vi "运维调试_总磷.vi"() -> ()   [LabVIEW 2016, in "斯坦道仪器.lvlib"]
uses:
  <vilib>/Utility/miscctls.llb/LVPointTypeDef.ctl
  <vilib>/Utility/config.llb/NI_LVConfig.lvlib
panel:
  in  "质控参数设置":bool
  out "字符串":string
  in  "总磷自动测试量程配置":T1
  out "温度2":sgl
  out "温度1":sgl
  out "ADC":sgl
  out "固件版本号":string
  in  "数组":string[](array[string])
  in  "备用系数写入":bool
  in  "备用系数读取":bool
  in  "备用系数":T2
  in  "量程切换阈值写入":bool
  in  "量程切换阈值读取":bool
  in  "量程切换阈值":cluster{"阈值":dbl, "标液浓度":dbl}
  in  "参数下拉列表":enum16{"总磷", "总氮"}(ring)
  in  "量程下拉列表":enum16{"低量程", "高量程"}(ring)
  in  "测量模式下拉列表":enum16{"水样测量", "空白核查", "跨度核查", "标样核查", "加标回收"}(ring)
  in  "公式":cluster{"X^2":dbl, "X":dbl, "b":dbl}
  in  "写公式":bool
  in  "读公式":bool
  in  "精度":dbl=4.0
  in  "样品5 F0":dbl
  in  "样品5 F1":dbl
  in  "样品4 F1":dbl
  in  "样品4 F0":dbl
  in  "样品3 F0":dbl
  in  "样品3 F1":dbl
  in  "样品2 F0":dbl
  in  "样品2 F1":dbl
  in  "样品1 F1":dbl
  in  "样品1 F0":dbl
  in  "method":u16(ring) items=["最小二乘", "最小绝对残差", "Bisquare"]
  in  "模型":enum32{"线性", "多项式"}(ring)
  out "r^2":dbl format="%.7g"
  out "拟合公式":string
  in  "样品2启用":bool
  in  "样品5启用":bool
  in  "样品4启用":bool
  in  "样品3启用":bool
  in  "样品1启用":bool
  in  "标液浓度5":dbl
  in  "测量吸光度5":dbl
  in  "标液浓度4":dbl
  in  "测量吸光度4":dbl
  in  "标液浓度3":dbl
  in  "测量吸光度3":dbl
  in  "标液浓度2":dbl
  in  "测量吸光度2":dbl
  in  "测量吸光度1":dbl
  in  "标液浓度1":dbl
  out "XY图":cluster{"X Values":dbl[], "Y Values":dbl[]}[](graph)
  in  "返回":bool
  in  "设置":bool
  out "序列号":string="序列号"
  out "总磷测量数据":T3(xcontrol)
  out "集成报警信息":string
  out "定时启动":bool
  out "总磷总氮运行状态":T4(xcontrol)
  in  "停止":bool
  in  "手动启动":bool
  in  "单步测试":bool
  in  "总磷氨氮调试":u16[](xcontrol)
  out "F3":sgl format="%#.6f"
  out "F2":sgl format="%#.6f"
  out "F1":sgl format="%#.6f"
  out "F0":sgl format="%#.6f"
  out "多列列表框":i32(listbox)
  # "参数设置"
  # "标液浓度"
  # "F0"
  # "F1"
  # "吸光值显示"
  # "样品一"
  # "辅\n助\n计\n算\n区"
  # "样品二"
  # "样品三"
  # "样品四"
  # "样品五"
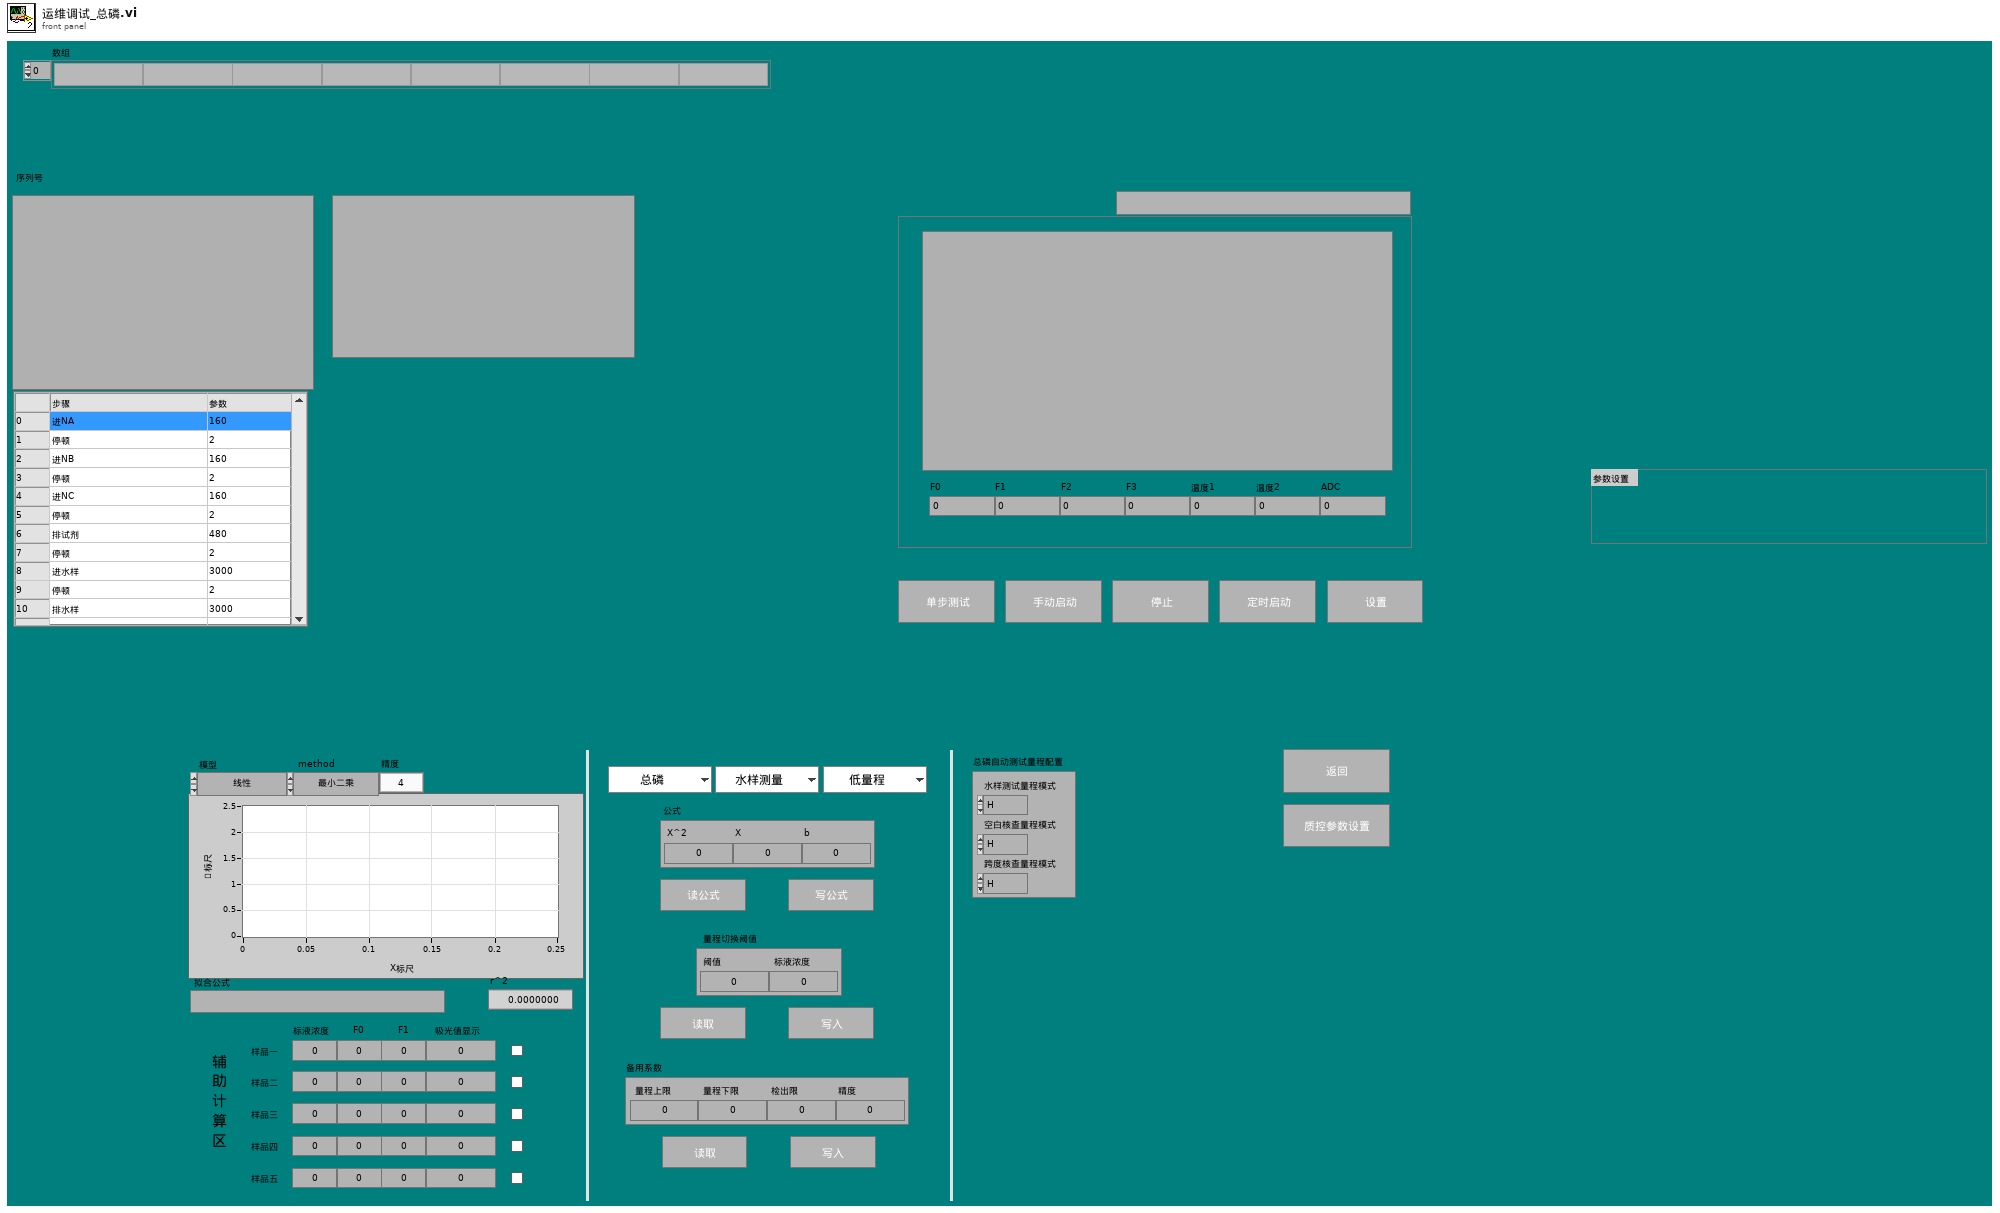
[diagram p1: front panel]
types:
  T1 = cluster{"水样测试量程模式":enum16{"H", "L", "AUTO"}, "空白核查量程模式":enum16{"H", "L", "AUTO"}, "跨度核查量程模式":enum16{"H", "L", "AUTO"}}
  T2 = cluster{"量程上限":dbl, "量程下限":dbl, "检出限":dbl, "精度":dbl}
  T3 = cluster{"flowid":u16, "测量精度":u16, "测量数据区":cluster{"因子编码":u32, "单位":u16, "标样参考值":sgl, "水样数据时间":timestamp, "水样实测值":sgl, "水样数据标识":string, "标样数据时间":timestamp, "标样实测值":sgl, "标样数据标识":string, "空白数据时间":timestamp, "空白实测值":sgl, "空白数据标识":string, "零点核查数据时间":timestamp, "零点核查实测值":sgl, "零点核查数据标识":string, "跨度核查数据时间":timestamp, "跨度核查实测值":sgl, "跨度核查数据标识":string, "加标回收数据时间":timestamp, "加标回收实测值":sgl, "加标回收数据标识":string, "平行样数据时间":timestamp, "平行样实测值":sgl, "平行样数据标识":string, "F0":sgl, "F1":sgl, "F2":sgl, "F3":sgl, "F4":sgl, "F5":sgl, "F6":sgl, "F7":sgl, "温度":sgl, "湿度":sgl, "X值":sgl}}
  T4 = cluster{"系统时间":timestamp, "工作状态":enum16{"空闲", "水样测试", "标样核查", "零点核查", "跨度核查", "空白测试", "平行样测试", "加标回收", "空白校准", "标样校准", "初始化（清洗）"}, "测量模式":enum16{"待机", "连续模式", "周期模式", "定点模式", "受控模式", "手动模式"}, "告警代码":enum16{"无告警", "缺试剂告警", "缺水样告警", "缺蒸馏水告警", "缺标液告警", "仪表漏液告警", "标定异常告警", "超量程告警", "加热异常", "低试剂预警", "超上限告警", "超下限告警", "仪表内部其他异常", "滴定异常告警", "电极异常告警", "量程切换告警", "参数设置告警", "PH电极电位异常", "电导率电极异常", "浊度光度异常", "溶解氧电极异常", "溶解氧光强异常", "温度异常告警", "PH异常告警", "溶解氧异常告警", "电导率异常告警", "浊度异常告警", "叶绿素异常告警", "藻密度异常告警", "蓝绿藻异常告警", "ORP异常告警", "氨氮异常告警", "清洁刷异常告警", "SD卡异常告警", "蓝牙异常告警", "Wifi异常告警", "流程异常告警"}, "故障代码":enum16{"无故障", "电机故障", "温度故障", "通讯故障", "滴定故障"}, "日志代码":u16, "软件版本":u16, "F0":sgl, "F1":sgl, "F2":sgl, "F3":sgl, "T":sgl, "H":sgl, "id":u16, "flowid":u16, "量程":u16, "总磷控温温度1":sgl, "营养盐控温温度2":sgl, "ADC":sgl}
  T5 = cluster{"站号":u16, "量程切换":enum32{"H", "L", "AUTO"}, "控制命令":enum16{"启动测量", "标样核查", "零点核查", "跨度核查", "空白测试", "平行样测试", "加标回收", "空白校准", "标样校准", "初始化（清洗）", "停止测试", "仪器重启", "校时", "模式设置", "测量间隔设置"}, "模式设置":enum16{"待机", "连续模式", "周期模式", "定点模式", "受控模式", "手动模式"}, "测量间隔":u16}
  T6 = enum16{"启动测量", "标样核查", "零点核查", "跨度核查", "空白测试", "平行样测试", "加标回收", "空白校准", "标样校准", "初始化（清洗）", "停止测试", "仪器重启", "校时", "模式设置", "测量间隔设置"}
  T7 = cluster{"仪器测试类型":enum16{"水样测试", "标样核查", "空白测试", "跨度核查"}, "周期设置类型":enum16{"定点启动", "间隔启动"}, "定时功能启用":bool, "定时间隔":dbl, "24H周期设置":bool[]}
  T8 = enum32{"Bad", "Idle", "Run top level", "Running"}
  T9 = typedef "LVDateTimeRec.ctl" = cluster{"秒数的小数部分":dbl, "秒":i32, "分":i32, "时":i32, "日":i32, "月":i32, "年":i32, "天数（周）":i32, "天数（年）":i32, "DST":i32}
  T10 = typedef "LVPointTypeDef.ctl" = cluster{"Horizontal":i16, "Vertical":i16}
  T11 = cluster{"因子编码":u32, "单位":u16, "标样参考值":sgl, "水样数据时间":timestamp, "水样实测值":sgl, "水样数据标识":string, "标样数据时间":timestamp, "标样实测值":sgl, "标样数据标识":string, "空白数据时间":timestamp, "空白实测值":sgl, "空白数据标识":string, "零点核查数据时间":timestamp, "零点核查实测值":sgl, "零点核查数据标识":string, "跨度核查数据时间":timestamp, "跨度核查实测值":sgl, "跨度核查数据标识":string, "加标回收数据时间":timestamp, "加标回收实测值":sgl, "加标回收数据标识":string, "平行样数据时间":timestamp, "平行样实测值":sgl, "平行样数据标识":string, "F0":sgl, "F1":sgl, "F2":sgl, "F3":sgl, "F4":sgl, "F5":sgl, "F6":sgl, "F7":sgl, "温度":sgl, "湿度":sgl, "X值":sgl}
  T12 = enum16{"空闲", "水样测试", "标样核查", "零点核查", "跨度核查", "空白测试", "平行样测试", "加标回收", "空白校准", "标样校准", "初始化（清洗）"}
  T13 = cluster{"启动模式":enum16{"标液测量", "水样测量", "零液测量", "盲样测量", "加标回收"}, "启动参数":u16, "量程":enum16{"低量程", "高量程"}}
  T14 = cluster{"时间标识":timestamp, "设备":string, "日志信息":string, "流程参数":string}
  T15 = cluster{"时间标识":timestamp, "设备":string, "日志信息":string}
  T16 = enum16{"无告警", "缺试剂告警", "缺水样告警", "缺蒸馏水告警", "缺标液告警", "仪表漏液告警", "标定异常告警", "超量程告警", "加热异常", "低试剂预警", "超上限告警", "超下限告警", "仪表内部其他异常", "滴定异常告警", "电极异常告警", "量程切换告警", "参数设置告警", "PH电极电位异常", "电导率电极异常", "浊度光度异常", "溶解氧电极异常", "溶解氧光强异常", "温度异常告警", "PH异常告警", "溶解氧异常告警", "电导率异常告警", "浊度异常告警", "叶绿素异常告警", "藻密度异常告警", "蓝绿藻异常告警", "ORP异常告警", "氨氮异常告警", "清洁刷异常告警", "SD卡异常告警", "蓝牙异常告警", "Wifi异常告警", "流程异常告警"}
  T17 = typedef "LVRowAndColumnUnsignedTypeDef.ctl" = cluster{"Row":u32, "Column":u32}
  T18 = typedef "NI_LVConfig.lvlib/Config Data RefNum.ctl" = refnum<k1>
  T19 = cluster{"XY图":cluster{"X Values":dbl[], "Y Values":dbl[]}[], "标液浓度1":dbl, "测量吸光度1":dbl, "测量吸光度2":dbl, "标液浓度2":dbl, "测量吸光度3":dbl, "标液浓度3":dbl, "测量吸光度4":dbl, "标液浓度4":dbl, "测量吸光度5":dbl, "标液浓度5":dbl, "样品1启用":bool, "样品3启用":bool, "样品4启用":bool, "样品5启用":bool, "样品2启用":bool, "拟合公式":string, "r^2":dbl, "模型":enum32{"线性", "多项式"}, "method":u16, "样品1 F0":dbl, "样品1 F1":dbl, "样品2 F1":dbl, "样品2 F0":dbl, "样品3 F1":dbl, "样品3 F0":dbl, "样品4 F0":dbl, "样品4 F1":dbl, "样品5 F1":dbl, "样品5 F0":dbl, "精度":dbl}
  T20 = cluster{"跨度值":dbl, "零点标准液浓度":dbl, "跨度标准液浓度":dbl, "标准液标准浓度":dbl}
  T21 = cluster{"确定":bool, "跨度值":dbl, "零点标准液浓度":dbl, "跨度标准液浓度":dbl, "标准液标准浓度":dbl}
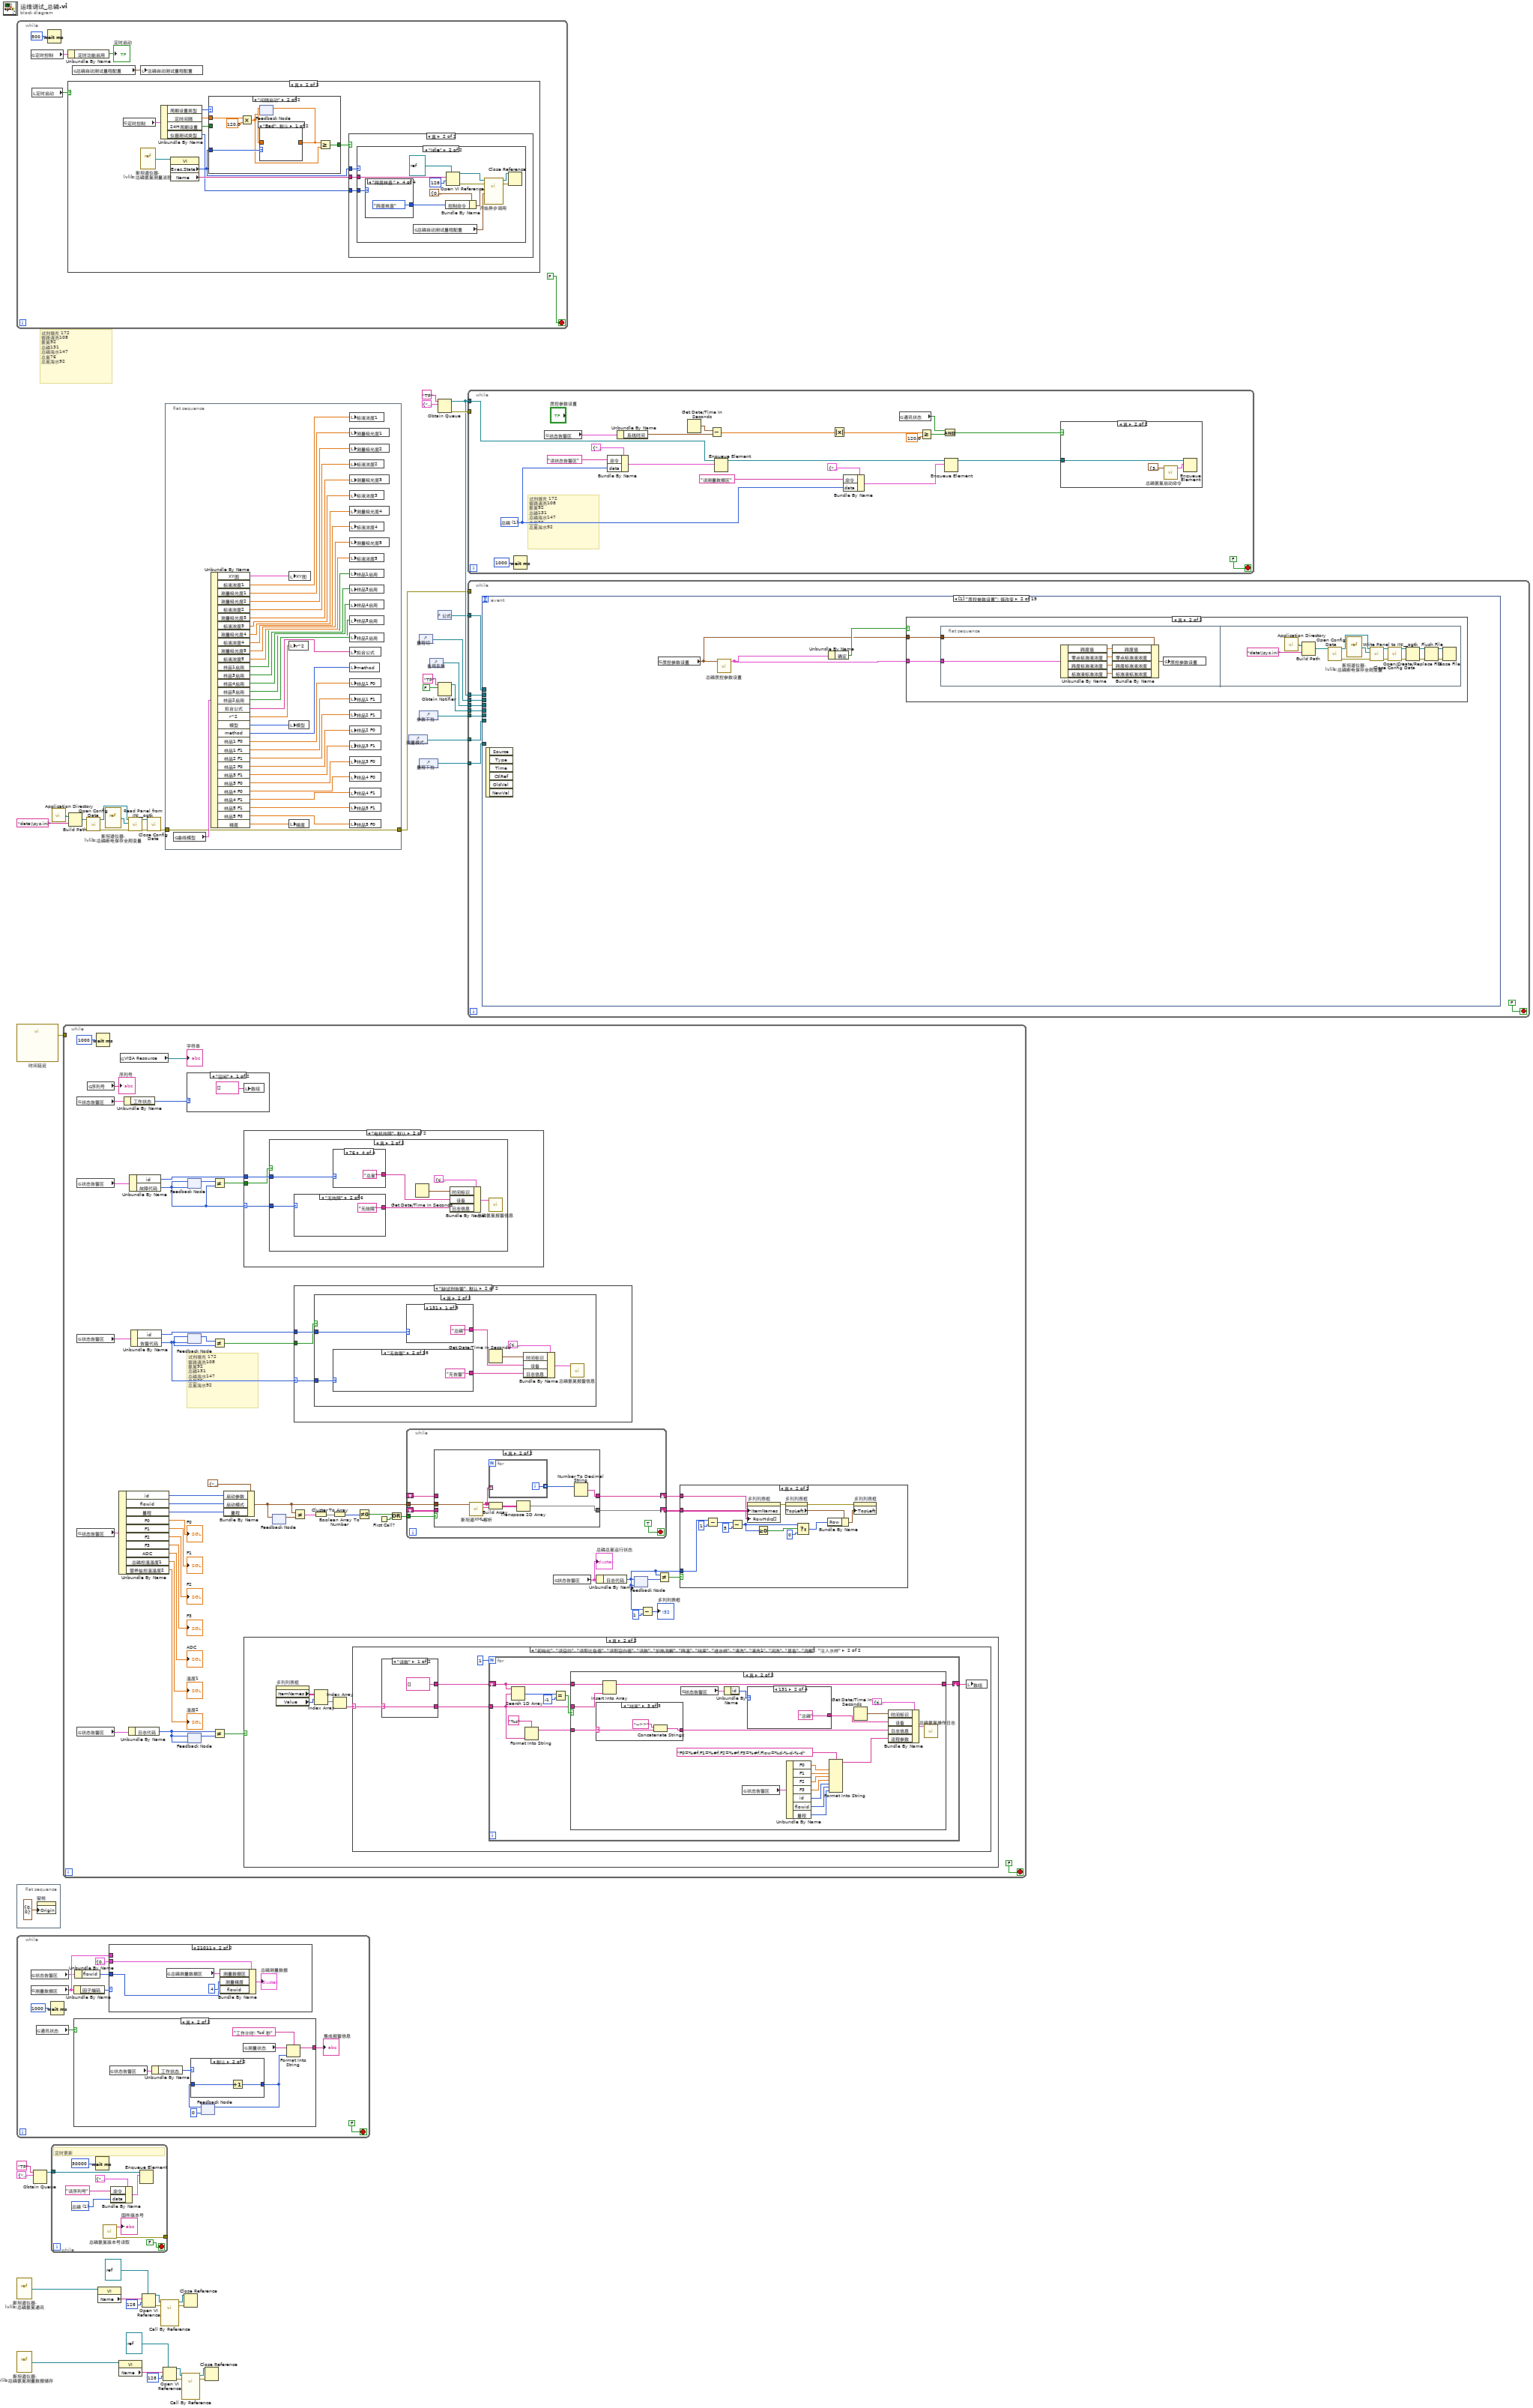
[diagram p0: block diagram]
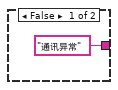
[diagram p2: hidden frame]
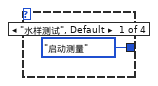
[diagram p8: hidden frame]
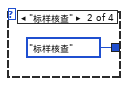
[diagram p9: hidden frame]
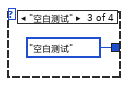
[diagram p10: hidden frame]
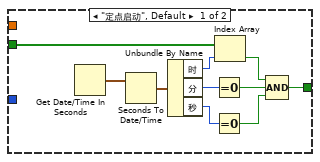
[diagram p11: hidden frame]
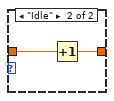
[diagram p12: hidden frame]
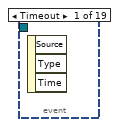
[diagram p13: hidden frame]
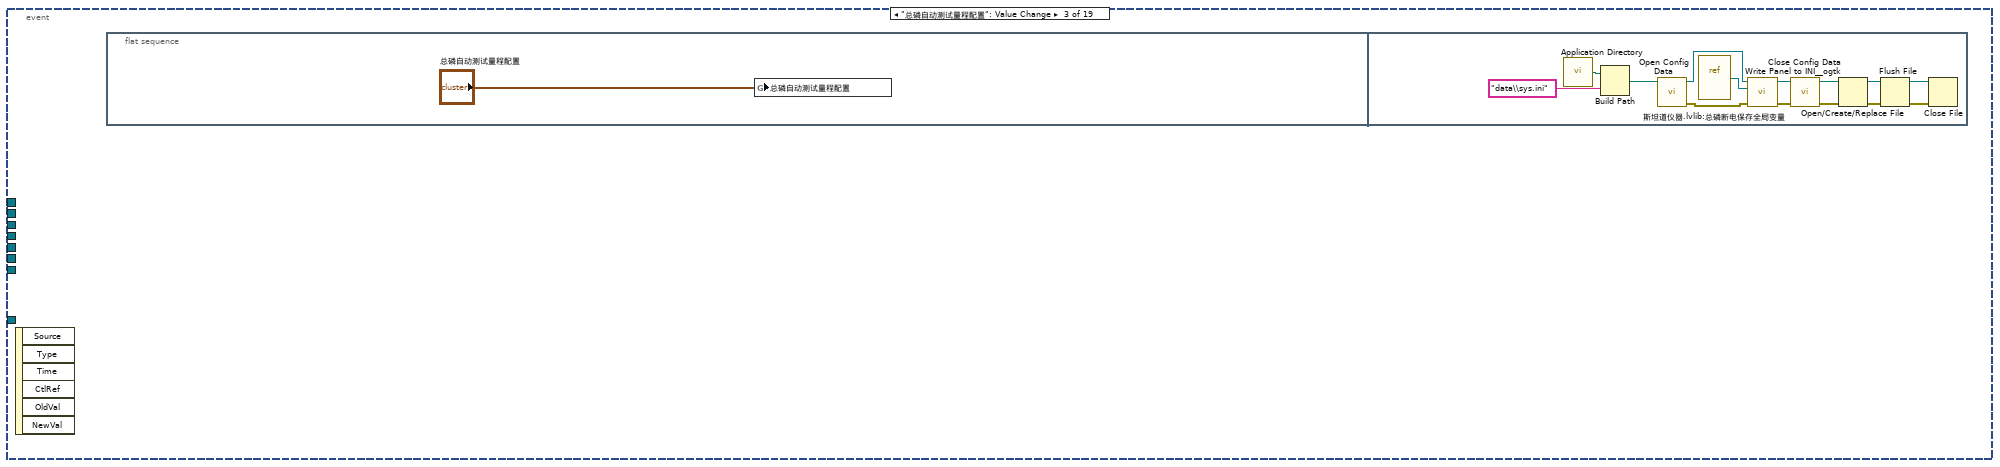
[diagram p15: hidden frame]
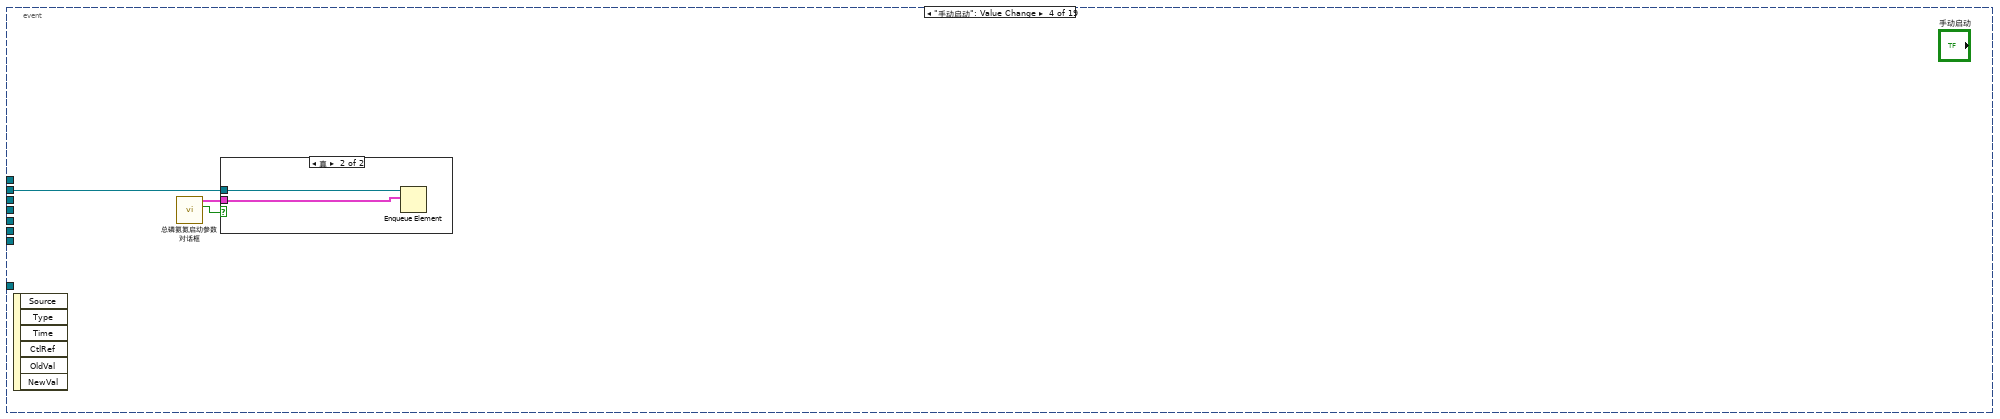
[diagram p16: hidden frame]
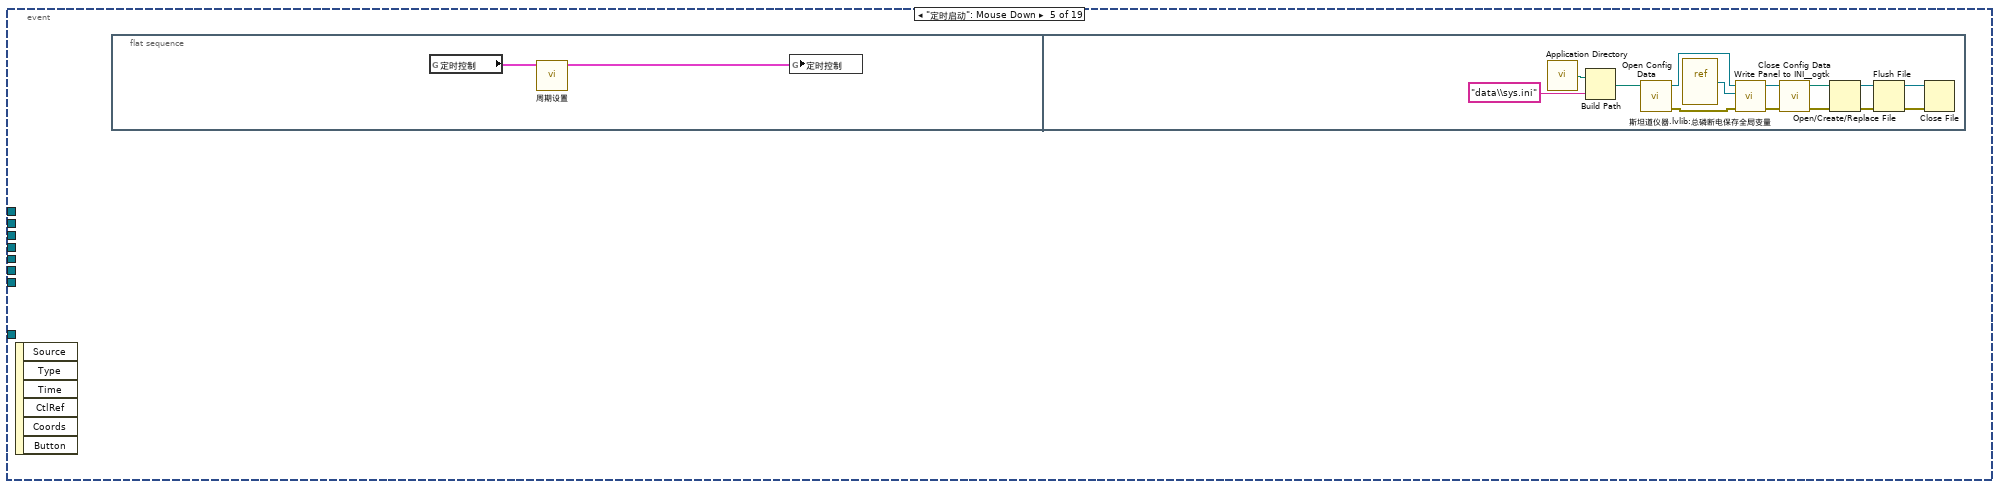
[diagram p18: hidden frame]
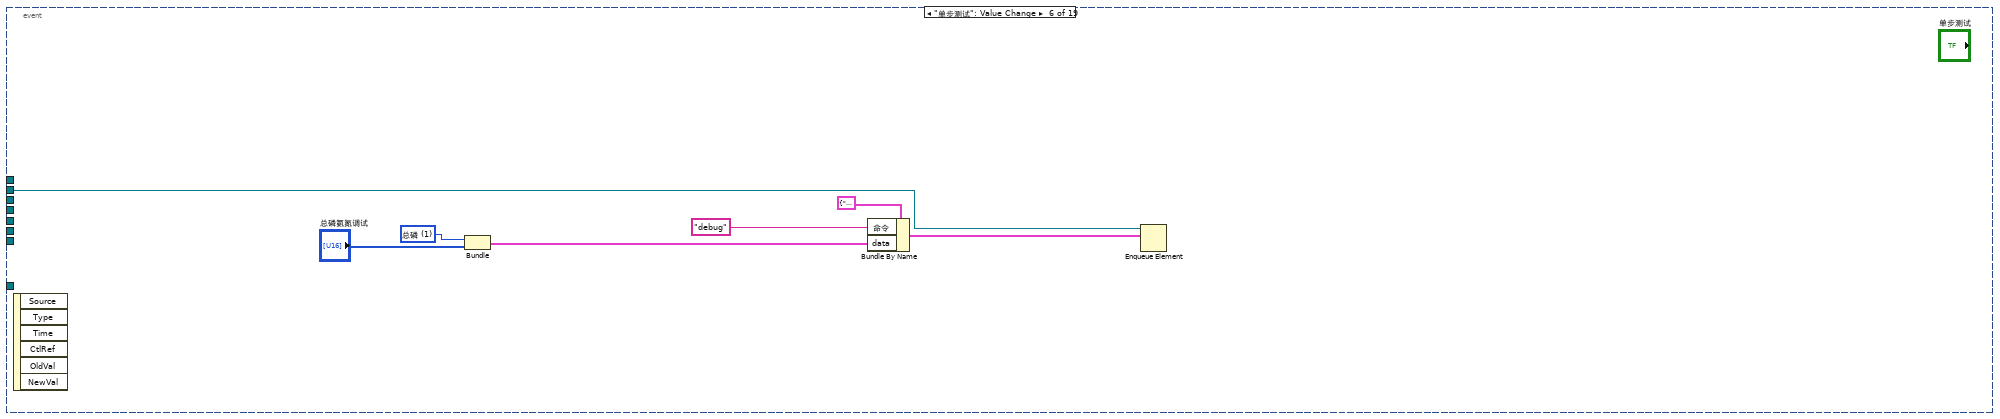
[diagram p19: hidden frame]
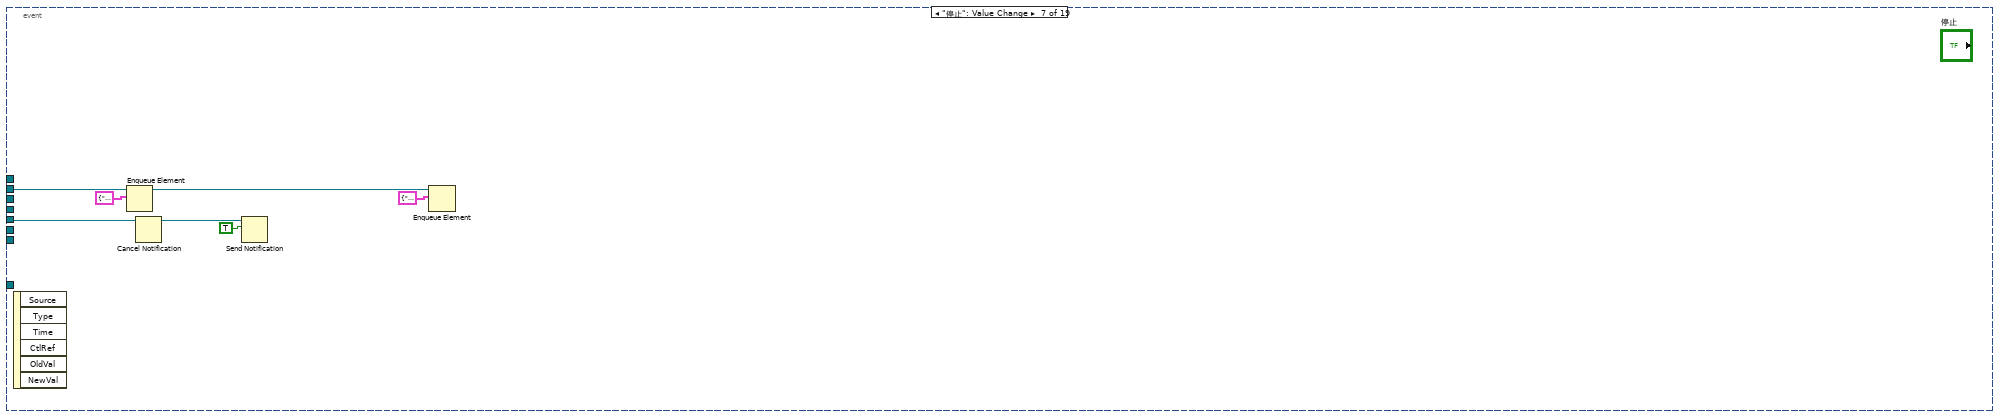
[diagram p20: hidden frame]
diagram:
  # "试剂填充 172 \n管路清洗108\n氨氮92\n总磷131\n总磷海水147\n总氮76\n总氮海水92"
  n1 = while {
    stop <- FALSE stop-if-true
    n2 = global read "总磷断电保存全局变量.vi" "定时控制"() -> (w46:T7)
    n3 = local read "定时启动"() -> (w47:bool)
    n4 = Wait (ms)(milliseconds to wait=u32 500 ("等待时间（毫秒）")) -> ()  [unwired: 1 out]
    n5 = Unbundle By Name(w46) -> ("定时功能启用"=→"定时启动":bool)
    n6 = case shown="真" w47 {
      frame False {
      }
      frame True {
        n7 = global read "总磷断电保存全局变量.vi" "定时控制"() -> (w51:T7)
        n8 = vi-ref "斯坦道仪器.lvlib:总磷氨氮测量流程.vi"() -> (w55:refnum<vi>)
        n9 = Unbundle By Name(w51) -> ("周期设置类型"=w58:enum16{"定点启动", "间隔启动"}, "定时间隔"=w57:dbl, "24H周期设置"=w56:bool[], "仪器测试类型"=w52:enum16{"水样测试", "标样核查", "空白测试", "跨度核查"})
        n10 = property class="VI"(reference=w55) -> ("Exec.State"=w50:T8, "Name"=w54:string)  [unwired: 1 in, 2 out]
        n11 = case shown="\"间隔启动\"" w58 {
          tunnel: w57 -> [_ w91]
          tunnel: w56 -> [w87 _]
          tunnel: w50 -> [_ w94]
          tunnel: [w86 w89] -> w53
          frame "定点启动", Default {
            n12 = Get Date/Time In Seconds() -> (seconds since 1Jan1904=w85:timestamp)
            n13 = Seconds To Date/Time(time stamp (now)=w85) -> (date time rec=w84:T9)  [unwired: 1 in]
            n14 = Unbundle By Name(w84) -> ("时"=w83:i32, "分"=w81:i32, "秒"=w82:i32)
            n15 = Equal To 0?(x=w81) -> (x = 0?=w79:bool)
            n16 = Equal To 0?(x=w82) -> (x = 0?=w78:bool)
            n17 = Index Array(array=w87, index=w83) -> (element=w80:bool)
            n18 = Compound Arithmetic op=AND ("复合运算")(w80, w79, w78) -> (w86:bool)
          }
          frame "间隔启动" {
            n19 = Multiply(x=w91, y=120.0) -> (x*y=w88:dbl)
            n20 = feedback #1(w88) -> (w93:dbl)
            n21 = case shown="\"Bad\", 默认" w94 {
              tunnel: w93 -> [_ w96]
              tunnel: [_ w95] -> w92
              frame "Bad", Default {
              }
              frame "Idle" {
                n22 = Increment(x=w96) -> (x+1=w95:dbl)
              }
            }
            n23 = feedback-in #1(w92) -> ()
            n24 = Greater Or Equal?(x=w92, y=w88) -> (x >= y?=w89:bool)
          }
        }
        n25 = case shown="真" w53 {
          tunnel: w54 -> [_ w61]
          tunnel: w52 -> [_ w60]
          tunnel: w50 -> [_ w59]
          frame False {
          }
          frame True {
            n26 = case shown="\"Idle\"" w59 {
              tunnel: w61 -> [_ w69]
              tunnel: w60 -> [_ w65]
              frame "Bad", Default {
              }
              frame "Idle" {
                n27 = case shown="\"跨度核查\"" w65 {
                  tunnel: [T6."启动测量" ("控制命令") T6."标样核查" ("控制命令") T6."空白测试" ("控制命令") T6."跨度核查" ("控制命令")] -> w64
                  frame "水样测试", Default {
                  }
                  frame "标样核查" {
                  }
                  frame "空白测试" {
                  }
                  frame "跨度核查" {
                  }
                }
                n28 = global read "总磷断电保存全局变量.vi" "总磷自动测试量程配置"() -> (w62:T1)
                n29 = Bundle By Name(cluster=T5 {"站号"=0, "量程切换"=enum."H", "控制命令"=enum."启动测量", "模式设置"=enum."待机", "测量间隔"=0} ("参数"), "控制命令"=w64) -> (w66:T5)
                n30 = Open VI Reference(type specifier VI Refnum (for type only)=refnum<vi> refnum, vi path=w69, options=128 ("选项")) -> (vi reference=w70:refnum<vi>, error out=w71:errorcluster)  [unwired: 3 in]
                n31 = call-by-ref "开始异步调用"(reference=w70, error in=w71, "量程模式"=w62, "参数"=w66) -> (reference out=w72:refnum<vi>, error out=w73:errorcluster)  [unwired: 10 in]
                n32 = Close Reference(reference=w72, error in (no error)=w73) -> ()  [unwired: 1 out]
              }
            }
          }
        }
      }
    }
    n33 = global read "总磷断电保存全局变量.vi" "总磷自动测试量程配置"() -> (w44:T1)
    n34 = local write "总磷自动测试量程配置"(w44) -> ()
  }
  n35 = call "时间延迟"() -> ("error out"=w17:errorcluster)  [unwired: 11 in]
  n36 = flat-sequence {
    frame #0 {
      n37 = property on="窗格" class="Pane"("Origin"=T10 {"Horizontal"=0, "Vertical"=0} ("原点")) -> ()  [unwired: 2 in, 2 out]
    }
  }
  n38 = while {
    stop <- FALSE stop-if-true
    n39 = global read "VAR总磷氨氮全局变量.vi" "状态告警区"() -> (w100:T4)
    n40 = global read "VAR总磷氨氮全局变量.vi" "测量数据区"() -> (w104:T11)
    n41 = global read "VAR总磷氨氮全局变量.vi" "通讯状态"() -> (w102:bool)
    n42 = Wait (ms)(milliseconds to wait=u32 1000 ("等待时间（毫秒）")) -> ()  [unwired: 1 out]
    n43 = Unbundle By Name(w104) -> ("因子编码"=w103:u32)
    n44 = case shown="真" w102 {
      tunnel: ["通讯异常" ("集成报警信息") w109] -> w101
      frame False {
      }
      frame True {
        n45 = global read "VAR总磷氨氮全局变量.vi" "状态告警区"() -> (w115:T4)
        n46 = Unbundle By Name(w115) -> ("工作状态"=w114:T12)
        n47 = feedback #2(0) -> (w112:i32)
        n48 = case shown="默认" w114 {
          tunnel: w112 -> [_ w117]
          tunnel: [_ w116] -> w110
          frame "空闲" {
          }
          frame Default {
            n49 = Increment(x=w117) -> (x+1=w116:i32)
          }
        }
        n50 = feedback-in #2(w110) -> ()
        n51 = global read "VAR总磷氨氮全局变量.vi" "测量状态"() -> (w108:string)
        n52 = Format Into String(format string="工作计时: %d 秒" ("格式字符串"), initial string=w108, w110) -> (resulting string=w109:string)  [unwired: 1 in, 1 out]
      }
    }
    "集成报警信息" <- w101
    n53 = Unbundle By Name(w100) -> ("flowid"=w99:u16)
    n54 = case shown="21011" w103 {
      tunnel: w104 -> [_ _]
      tunnel: w99 -> [_ w120]
      tunnel: T3 {"flowid"=0, "测量精度"=0, "测量数据区"={"因子编码"=0, "单位"=0, "标样参考值"=0.0, "水样数据时间"=timestamp(0 s since 1904-01-01), "水样实测值"=0.0, "水样数据标识"="", "标样数据时间"=timestamp(0 s since 1904-01-01), "标样实测值"=0.0, "标样数据标识"="", "空白数据时间"=timestamp(0 s since 1904-01-01), "空白实测值"=0.0, "空白数据标识"="", "零点核查数据时间"=timestamp(0 s since 1904-01-01), "零点核查实测值"=0.0, "零点核查数据标识"="", "跨度核查数据时间"=timestamp(0 s since 1904-01-01), "跨度核查实测值"=0.0, "跨度核查数据标识"="", "加标回收数据时间"=timestamp(0 s since 1904-01-01), "加标回收实测值"=0.0, "加标回收数据标识"="", "平行样数据时间"=timestamp(0 s since 1904-01-01), "平行样实测值"=0.0, "平行样数据标识"="", "F0"=0.0, "F1"=0.0, "F2"=0.0, "F3"=0.0, "F4"=0.0, "F5"=0.0, "F6"=0.0, "F7"=0.0, "温度"=0.0, "湿度"=0.0, "X值"=0.0}} ("总氮测量数据") -> [_ w119]
      frame Default {
      }
      frame 21011 {
        n55 = global read "VAR总磷氨氮全局变量.vi" "总磷测量数据区"() -> (w118:T11)
        n56 = Bundle By Name(cluster=w119, "测量数据区"=w118, "测量精度"=u16 4, "flowid"=w120) -> (→"总磷测量数据":T3)
      }
    }
  }
  n57 = vi-ref "斯坦道仪器.lvlib:总磷氨氮通讯.vi"() -> (w39:refnum<vi>)
  n58 = vi-ref "斯坦道仪器.lvlib:总磷氨氮测量数据储存.vi"() -> (w31:refnum<vi>)
  n59 = Obtain Queue(name (unnamed)="TP" ("名称（未命名）"), element data type=cluster{"命令":string, "data":variant} {"命令"="", "data"=variant}) -> (queue out=w14:refnum<queue>)  [unwired: 3 in, 2 out]
  n60 = while {
    tunnel: w14 -> [w128]
    tunnel: [w124] -> _
    stop <- FALSE stop-if-true
    w125 = u16 1 items=["总磷"=1, "总氮"=2, "氨氮"=3] ("站号")
    # "定时更新"
    n61 = Wait (ms)(milliseconds to wait=u32 30000 ("等待时间（毫秒）")) -> ()  [unwired: 1 out]
    n62 = call "总磷氨氮版本号读取.vi"() -> ("error out"=w124:errorcluster, "固件版本号"=→"固件版本号":string)  [unwired: 10 in]
    n63 = Bundle By Name(cluster=cluster{"命令":string, "data":variant} {"命令"="", "data"=variant} ("元素"), "命令"="读序列号", "data"=w125) -> (w127:cluster{"命令":string, "data":variant})
    n64 = Enqueue Element(queue=w128, element=w127) -> ()  [unwired: 2 in, 3 out]
  }
  n65 = call <vilib>:"Application Directory.vi"() -> ("Application Directory"=w3:path)
  n66 = while {
    tunnel: w17 -> [_]
    stop <- FALSE stop-if-true
    # "试剂填充 172 \n管路清洗108\n氨氮92\n总磷131\n总磷海水147\n总氮76\n总氮海水92"
    n67 = global read "VAR总磷氨氮全局变量.vi" "状态告警区"() -> (w144:T4)
    n68 = global read "VAR总磷氨氮全局变量.vi" "状态告警区"() -> (w149:T4)
    n69 = global read "VAR总磷氨氮全局变量.vi" "状态告警区"() -> (w154:T4)
    n70 = global read "VAR总磷氨氮全局变量.vi" "状态告警区"() -> (w166:T4)
    n71 = global read "VAR总磷氨氮全局变量.vi" "状态告警区"() -> (w141:T4)
    n72 = global read "VAR总磷氨氮全局变量.vi" "序列号"() -> (→"序列号":string)
    n73 = Wait (ms)(milliseconds to wait=u32 1000 ("等待时间（毫秒）")) -> ()  [unwired: 1 out]
    n74 = Unbundle By Name(w166) -> ("id"=w163:u16, "flowid"=w165:u16, "量程"=w164:u16, "F0"=→"F0":sgl, "F1"=→"F1":sgl, "F2"=→"F2":sgl, "F3"=→"F3":sgl, "ADC"=→"ADC":sgl, "总磷控温温度1"=→"温度1":sgl, "营养盐控温温度2"=→"温度2":sgl)
    n75 = global read "VAR总磷氨氮全局变量.vi" "VISA Resource"() -> (→"字符串":refnum<visa-resource-name>)
    n76 = Unbundle By Name(w144) -> ("工作状态"=w143:T12)
    n77 = Unbundle By Name(w141) -> ("日志代码"=w140:u16)
    n78 = Unbundle By Name(w149) -> ("id"=w148:u16, "故障代码"=w145:enum16{"无故障", "电机故障", "温度故障", "通讯故障", "滴定故障"})
    n79 = Unbundle By Name(w154) -> ("id"=w153:u16, "告警代码"=w150:T16)
    n80 = case shown="\"空闲\"" w143 {
      frame "空闲" {
        n81 = local write "数组"(string[] [] ("数组")) -> ()
      }
      frame "水样测试", Default {
      }
    }
    n82 = feedback #3(w145) -> (w146:enum16{"无故障", "电机故障", "温度故障", "通讯故障", "滴定故障"})
    n83 = feedback-in #3(w145) -> ()
    n84 = feedback #4(w150) -> (w151:T16)
    n85 = feedback-in #4(w150) -> ()
    n86 = feedback #5(w140) -> (w142:u16)
    n87 = feedback-in #5(w140) -> ()
    n88 = Not Equal?(x=w146, y=w145) -> (x != y?=w147:bool)
    n89 = Not Equal?(x=w151, y=w150) -> (x != y?=w152:bool)
    n90 = Not Equal?(x=w140, y=w142) -> (x != y?=w139:bool)
    n91 = Bundle By Name(cluster=T13 {"启动模式"=enum."加标回收", "启动参数"=1, "量程"=enum."低量程"} ("参数簇"), "启动参数"=w163, "启动模式"=w165, "量程"=w164) -> (w156:T13)
    n92 = case shown="\"电机故障\", 默认" w145 {
      selector: w145 -> [_ w235]
      tunnel: w148 -> [_ w236]
      tunnel: w147 -> [_ w234]
      frame "无故障" {
      }
      frame "电机故障", Default {
        n93 = case shown="真" w234 {
          tunnel: w236 -> [_ w243]
          tunnel: w235 -> [_ w238]
          frame False {
          }
          frame True {
            n94 = case shown="\"无故障\"" w238 {
              selector: w238 -> [w245 _ _ _ _ _]
              tunnel: [w244 "无故障" "电机故障" "温度故障" "通讯故障" "滴定故障"] -> w237
              frame Default {
                n95 = Format Into String(format string="%d" ("格式字符串"), initial string="未知" ("工作状态"), w245) -> (resulting string=w244:string)  [unwired: 1 in, 1 out]
              }
              frame "无故障" {
              }
              frame "电机故障" {
              }
              frame "温度故障" {
              }
              frame "通讯故障" {
              }
              frame "滴定故障" {
              }
            }
            n96 = case shown="76" w243 {
              tunnel: [_ "总磷" ("table输入") "氨氮" ("table输入") "总氮" ("table输入")] -> w239
              frame Default {
              }
              frame 131 {
              }
              frame 92 {
              }
              frame 76 {
              }
            }
            n97 = Get Date/Time In Seconds() -> (seconds since 1Jan1904=w240:timestamp)
            n98 = Bundle By Name(cluster=T15 {"时间标识"=timestamp(0 s since 1904-01-01), "设备"="", "日志信息"=""} ("data in"), "时间标识"=w240, "设备"=w239, "日志信息"=w237) -> (w241:T15)
            n99 = call "总磷氨氮报警信息.vi"("data in"=w241) -> ()  [unwired: 11 in]
          }
        }
      }
    }
    n100 = case shown="真" w139 {
      frame False {
      }
      frame True {
        n101 = property on="多列列表框" class="MCListbox (严格)"() -> ("ItemNames"=w183:string[][], "Value"=w184:i32)  [unwired: 2 in, 2 out]
        n102 = Index Array(array=w183, index (row)=w184) -> (element=w182:string[])  [unwired: 1 in]
        n103 = Index Array(array=w182) -> (element=w181:string)  [unwired: 1 in]
        n104 = case shown="\"初始化\", \"读空白\", \"读取比色值\", \"读取空白值\", \"读数\", \"加热消解\", \"降温\", \"结束\", \"进水样\", \"清洗\", \"清洗1\", \"润洗\", \"显色\", \"消解\", \"注入水样\"" w181 {
          selector: w181 -> [_ w187]
          frame Default {
          }
          frame "初始化", "读空白", "读取比色值", "读取空白值", "读数", "加热消解", "降温", "结束", "进水样", "清洗", "清洗1", "润洗", "显色", "消解", "注入水样" {
            n105 = case shown="\"读数\"" w187 {
              selector: w187 -> [w191 w193]
              tunnel: [w191 w193] -> w186
              tunnel: [string[] [] ("数组") "数组"] -> w185
              frame "读数" {
              }
              frame Default {
              }
            }
            n106 = for {
              N: 1 -> [_]
              tunnel: w186 -> [w195]
              shift-right: [w194] -> w188
              shift-left: w185 -> [w196]
              n107 = Search 1D Array(1D array=w196, element=w195) -> (index of element=w199:i32)  [unwired: 1 in]
              n108 = Format Into String(format string="%s" ("格式字符串"), w195) -> (resulting string=w200:string)  [unwired: 2 in, 1 out]
              n109 = Equal?(x=w199, y=-1) -> (x = y?=w197:bool)
              n110 = case shown="真" w197 {
                tunnel: w200 -> [_ w204]
                tunnel: w196 -> [w202 w208]
                tunnel: w195 -> [_ w207]
                tunnel: [w202 w206] -> w194
                frame False {
                }
                frame True {
                  n111 = case shown="\"结束\"" w204 {
                    selector: w204 -> [w224 w227 w230]
                    tunnel: [w224 w226 w229] -> w203
                    frame Default {
                    }
                    frame "初始化" {
                      n112 = Concatenate Strings("-->>" ("字符串"), w227) -> (w226:string)
                    }
                    frame "结束" {
                      n113 = Concatenate Strings("-->>" ("字符串"), w230) -> (w229:string)
                    }
                  }
                  n114 = Insert Into Array(array=w208, new element=w207) -> (w206:string[])  [unwired: 1 in]
                  n115 = global read "VAR总磷氨氮全局变量.vi" "状态告警区"() -> (w223:T4)
                  n116 = Unbundle By Name(w223) -> ("id"=w222:u16)
                  n117 = global read "VAR总磷氨氮全局变量.vi" "状态告警区"() -> (w218:T4)
                  n118 = case shown="131" w222 {
                    tunnel: [_ "总磷" ("table输入") "氨氮" ("table输入") "总氮" ("table输入")] -> w220
                    frame Default {
                    }
                    frame 131 {
                    }
                    frame 92 {
                    }
                    frame 76 {
                    }
                  }
                  n119 = Unbundle By Name(w218) -> ("F0"=w215:sgl, "F1"=w214:sgl, "F2"=w213:sgl, "F3"=w212:sgl, "id"=w211:u16, "flowid"=w210:u16, "量程"=w209:u16)
                  n120 = Format Into String(format string="F0=%#f,F1=%#f,F2=%#f,F3=%#f,Flow=%d-%-d-%-d" ("格式字符串"), w215, w214, w213, w212, w211, w210, w209) -> (resulting string=w216:string)  [unwired: 2 in, 1 out]
                  n121 = Get Date/Time In Seconds() -> (seconds since 1Jan1904=w219:timestamp)
                  n122 = Bundle By Name(cluster=T14 {"时间标识"=timestamp(0 s since 1904-01-01), "设备"="", "日志信息"="", "流程参数"=""} ("data in"), "时间标识"=w219, "设备"=w220, "日志信息"=w203, "流程参数"=w216) -> (w221:T14)
                  n123 = call "总磷氨氮操作日志.vi"("data in"=w221) -> ()  [unwired: 11 in]
                }
              }
            }
            n124 = local write "数组"(w188) -> ()
          }
        }
      }
    }
    n125 = feedback #6() -> (w172:T13)  [unwired: 1 in]
    n126 = feedback-in #6(w156) -> ()
    n127 = Not Equal?(x=w156, y=w172) -> (x != y?=w173:cluster{"启动模式":bool, "启动参数":bool, "量程":bool})
    n128 = case shown="\"缺试剂告警\", 默认" w150 {
      selector: w150 -> [_ w257]
      tunnel: w153 -> [_ w258]
      tunnel: w152 -> [_ w256]
      frame "无告警" {
      }
      frame "缺试剂告警", Default {
        n129 = case shown="真" w256 {
          tunnel: w258 -> [_ w265]
          tunnel: w257 -> [_ w259]
          frame False {
          }
          frame True {
            n130 = case shown="\"无告警\"" w259 {
              selector: w259 -> [w267 _ _ _ _ _ _ _ _ _ _ _ _ _ _ _ _ _ _ _ _ _ _ _ _ _ _ _ _ _ _ _ _ _ _ _ _ _]
              tunnel: [w266 "无告警" "缺试剂告警" "缺水样告警" "缺蒸馏水告警" "缺标液告警" "仪表漏液告警" "标定异常告警" "超量程告警" "加热异常" "低试剂预警" "超上限告警" "超下限告警" "仪表内部其他异常" "滴定异常告警" "电极异常告警" "量程切换告警" "参数设置告警" "PH电极电位异常" "电导率电极异常" "浊度光度异常" "溶解氧电极异常" "溶解氧光强异常" "温度异常告警" "PH异常告警" "溶解氧异常告警" "电导率异常告警" "浊度异常告警" "叶绿素异常告警" "藻密度异常告警" "蓝绿藻异常告警" "ORP异常告警" "氨氮异常告警" "清洁刷异常告警" "SD卡异常告警" "蓝牙异常告警" "WiFi异常告警" "流程异常告警"] -> w260
              frame Default {
                n131 = Format Into String(format string="%d" ("格式字符串"), initial string="未知" ("工作状态"), w267) -> (resulting string=w266:string)  [unwired: 1 in, 1 out]
              }
              frame "无告警" {
              }
              frame "缺试剂告警" {
              }
              frame "缺水样告警" {
              }
              frame "缺蒸馏水告警" {
              }
              frame "缺标液告警" {
              }
              frame "仪表漏液告警" {
              }
              frame "标定异常告警" {
              }
              frame "超量程告警" {
              }
              frame "加热异常" {
              }
              frame "低试剂预警" {
              }
              frame "超上限告警" {
              }
              frame "超下限告警" {
              }
              frame "仪表内部其他异常" {
              }
              frame "滴定异常告警" {
              }
              frame "电极异常告警" {
              }
              frame "量程切换告警" {
              }
              frame "参数设置告警" {
              }
              frame "PH电极电位异常" {
              }
              frame "电导率电极异常" {
              }
              frame "浊度光度异常" {
              }
              frame "溶解氧电极异常" {
              }
              frame "溶解氧光强异常" {
              }
              frame "温度异常告警" {
              }
              frame "PH异常告警" {
              }
              frame "溶解氧异常告警" {
              }
              frame "电导率异常告警" {
              }
              frame "浊度异常告警" {
              }
              frame "叶绿素异常告警" {
              }
              frame "藻密度异常告警" {
              }
              frame "蓝绿藻异常告警" {
              }
              frame "ORP异常告警" {
              }
              frame "氨氮异常告警" {
              }
              frame "清洁刷异常告警" {
              }
              frame "SD卡异常告警" {
              }
              frame "蓝牙异常告警" {
              }
              frame "Wifi异常告警" {
              }
              frame "流程异常告警" {
              }
            }
            n132 = case shown="131" w265 {
              tunnel: ["总磷" ("table输入") "氨氮" ("table输入") "总氮" ("table输入")] -> w261
              frame 131 {
              }
              frame 92 {
              }
              frame 76, Default {
              }
            }
            n133 = Get Date/Time In Seconds() -> (seconds since 1Jan1904=w262:timestamp)
            n134 = Bundle By Name(cluster=T15 {"时间标识"=timestamp(0 s since 1904-01-01), "设备"="", "日志信息"=""} ("data in"), "时间标识"=w262, "设备"=w261, "日志信息"=w260) -> (w263:T15)
            n135 = call "总磷氨氮报警信息.vi"("data in"=w263) -> ()  [unwired: 11 in]
          }
        }
      }
    }
    n136 = Cluster To Array(cluster=w173) -> (array=w174:bool[])
    n137 = Boolean Array To Number(Boolean array=w174) -> (number=w175:u32)
    n138 = Not Equal To 0?(x=w175) -> (x != 0?=w168:bool)
    n139 = First Call?() -> (First Call?: T/F=w169:bool)
    n140 = Or(x=w168, y=w169) -> (x .or. y?=w167:bool)
    n141 = while {
      tunnel: w167 -> [w316]
      tunnel: w156 -> [w315]
      shift-right: [w314] -> w171
      shift-left: _ -> [w310]
      shift-right: [w313] -> w170
      shift-left: _ -> [w311]
      stop <- TRUE stop-if-true
      n142 = case shown="真" w316 {
        tunnel: [w318 w325] -> w313
        tunnel: [w317 w324] -> w314
        tunnel: w315 -> [_ w319]
        tunnel: w311 -> [w318 _]
        tunnel: w310 -> [w317 _]
        frame False {
        }
        frame True {
          n143 = call "斯坦道XML解析.vi"("参数簇"=w319) -> ("步骤时间"=w320:string[], "步骤名"=w322:string[])  [unwired: 9 in]
          n144 = for {
            tunnel: w322 -> [_] mode=indexing
            tunnel: [w326] -> w323 mode=indexing
            i -> [w326]
          }
          n145 = Build Array(w322, w320) -> (w321:string[][])
          n146 = Transpose 2D Array(2D array=w321) -> (transposed array=w324:string[][])
          n147 = Number To Decimal String(number=w323) -> (decimal integer string=w325:string[])  [unwired: 1 in]
        }
      }
    }
    n148 = global read "VAR总磷氨氮全局变量.vi" "状态告警区"() -> (w157:T4)
    "总磷总氮运行状态" <- w157
    n149 = Unbundle By Name(w157) -> ("日志代码"=w137:u16)
    n150 = feedback-in #7(w137) -> ()
    n151 = feedback #7(w137) -> (w177:u16)
    n152 = Subtract(x=w137, y=1) -> (x-y=→"多列列表框":i32)
    n153 = Not Equal?(x=w137, y=w177) -> (x != y?=w176:bool)
    n154 = case shown="真" w176 {
      tunnel: w137 -> [_ w329]
      tunnel: w171 -> [_ w336]
      tunnel: w170 -> [_ w335]
      frame False {
      }
      frame True {
        n155 = Subtract(x=w329, y=1) -> (x-y=w327:i32)
        n156 = Subtract(x=w327, y=5) -> (x-y=w331:i32)
        n157 = property on="多列列表框" class="MCListbox (严格)"("ItemNames"=w336, "RowHdrs[]"=w335) -> (error out=w337:errorcluster)  [unwired: 2 in, 1 out]
        n158 = Greater Or Equal To 0?(x=w331) -> (x >= 0?=w330:bool)
        n159 = property on="多列列表框" class="MCListbox (严格)"(error in=w337) -> (error out=w338:errorcluster, "TopLeft"=w339:T17)  [unwired: 1 in, 1 out]
        n160 = Select(t=w331, s=w330, f=0) -> (s? t:f=w332:i32)
        n161 = Bundle By Name(cluster=w339, "Row"=w332) -> (w340:T17)
        n162 = property on="多列列表框" class="MCListbox (严格)"(error in=w338, "TopLeft"=w340) -> ()  [unwired: 1 in, 2 out]
      }
    }
  }
  n163 = Build Path(base path=w3, name or relative path="data\\sys.ini" ("名称或相对路径")) -> (appended path=w5:path)
  n164 = call <vilib>:"Open Config Data.vi"("configuration file path"=w5) -> ("error out"=w9:errorcluster, "refnum"=w6:T18)  [unwired: 8 in, 1 out]
  n165 = property class="VI"(reference=w39) -> ("Name"=w38:string)  [unwired: 1 in, 2 out]
  n166 = vi-ref "斯坦道仪器.lvlib:总磷断电保存全局变量.vi"() -> (w7:refnum<vi>)
  n167 = property class="VI"(reference=w31) -> ("Name"=w24:string)  [unwired: 1 in, 2 out]
  n168 = call <userlib>:"Read Panel from INI__ogtk.vi"("error in (no error)"=w9, "VI ref"=w7, "refnum"=w6) -> ("error out"=w10:errorcluster, "refnum out"=w8:T18)  [unwired: 7 in]
  n169 = Open VI Reference(type specifier VI Refnum (for type only)=refnum<vi> refnum, vi path=w38, options=128 ("选项")) -> (vi reference=w36:refnum<vi>, error out=w34:errorcluster)  [unwired: 3 in]
  n170 = call <vilib>:"Close Config Data.vi"("error in (no error)"=w10, "refnum"=w8) -> ("error out"=w2:errorcluster)  [unwired: 8 in, 1 out]
  n171 = call-by-ref "?"(reference=w36, error in=w34) -> (reference out=w32:refnum<vi>, error out=w33:errorcluster)  [unwired: 12 in]
  n172 = Open VI Reference(type specifier VI Refnum (for type only)=refnum<vi> refnum, vi path=w24, options=128 ("选项")) -> (vi reference=w26:refnum<vi>, error out=w28:errorcluster)  [unwired: 3 in]
  n173 = flat-sequence {
    tunnel: w2 -> [w341]
    tunnel: [w341] -> w1
    frame #0 {
      n174 = global read "总磷断电保存全局变量.vi" "曲线模型"() -> (w373:T19)
      n175 = Unbundle By Name(w373) -> ("XY图"=w372:cluster{"X Values":dbl[], "Y Values":dbl[]}[], "标液浓度1"=w371:dbl, "测量吸光度1"=w370:dbl, "测量吸光度2"=w369:dbl, "标液浓度2"=w362:dbl, "测量吸光度3"=w368:dbl, "标液浓度3"=w363:dbl, "测量吸光度4"=w367:dbl, "标液浓度4"=w364:dbl, "测量吸光度5"=w366:dbl, "标液浓度5"=w365:dbl, "样品1启用"=w361:bool, "样品3启用"=w360:bool, "样品4启用"=w359:bool, "样品5启用"=w358:bool, "样品2启用"=w357:bool, "拟合公式"=w356:string, "r^2"=w355:dbl, "模型"=w354:enum32{"线性", "多项式"}, "method"=w353:u16, "样品1 F0"=w352:dbl, "样品1 F1"=w351:dbl, "样品2 F1"=w350:dbl, "样品2 F0"=w349:dbl, "样品3 F1"=w348:dbl, "样品3 F0"=w347:dbl, "样品4 F0"=w346:dbl, "样品4 F1"=w345:dbl, "样品5 F1"=w344:dbl, "样品5 F0"=w343:dbl, "精度"=w342:dbl)
      n176 = local write "XY图"(w372) -> ()
      n177 = local write "r^2"(w355) -> ()
      n178 = local write "模型"(w354) -> ()
      n179 = local write "精度"(w342) -> ()
      n180 = local write "标液浓度1"(w371) -> ()
      n181 = local write "测量吸光度1"(w370) -> ()
      n182 = local write "测量吸光度2"(w369) -> ()
      n183 = local write "标液浓度2"(w362) -> ()
      n184 = local write "测量吸光度3"(w368) -> ()
      n185 = local write "标液浓度3"(w363) -> ()
      n186 = local write "测量吸光度4"(w367) -> ()
      n187 = local write "标液浓度4"(w364) -> ()
      n188 = local write "测量吸光度5"(w366) -> ()
      n189 = local write "标液浓度5"(w365) -> ()
      n190 = local write "样品1启用"(w361) -> ()
      n191 = local write "样品3启用"(w360) -> ()
      n192 = local write "样品4启用"(w359) -> ()
      n193 = local write "样品5启用"(w358) -> ()
      n194 = local write "样品2启用"(w357) -> ()
      n195 = local write "拟合公式"(w356) -> ()
      n196 = local write "method"(w353) -> ()
      n197 = local write "样品1 F0"(w352) -> ()
      n198 = local write "样品1 F1"(w351) -> ()
      n199 = local write "样品2 F1"(w350) -> ()
      n200 = local write "样品2 F0"(w349) -> ()
      n201 = local write "样品3 F1"(w348) -> ()
      n202 = local write "样品3 F0"(w347) -> ()
      n203 = local write "样品4 F0"(w346) -> ()
      n204 = local write "样品4 F1"(w345) -> ()
      n205 = local write "样品5 F1"(w344) -> ()
      n206 = local write "样品5 F0"(w343) -> ()
    }
  }
  n207 = call-by-ref "?"(reference=w26, error in=w28) -> (reference out=w30:refnum<vi>, error out=w29:errorcluster)  [unwired: 12 in]
  n208 = Close Reference(reference=w32, error in (no error)=w33) -> ()  [unwired: 1 out]
  n209 = Close Reference(reference=w30, error in (no error)=w29) -> ()  [unwired: 1 out]
  n210 = control-ref of="测量模式下拉列表"() -> (w21:refnum<vi>)
  n211 = control-ref of="量程切换阈值"() -> (w19:refnum<vi>)
  n212 = control-ref of="参数下拉列表"() -> (w22:refnum<vi>)
  n213 = control-ref of="量程下拉列表"() -> (w23:refnum<vi>)
  n214 = control-ref of="备用系数"() -> (w18:refnum<vi>)
  n215 = control-ref of="公式"() -> (w20:refnum<vi>)
  n216 = Obtain Queue(name (unnamed)="TP" ("名称（未命名）"), element data type=cluster{"命令":string, "data":variant} {"命令"="", "data"=variant}) -> (queue out=w40:refnum<queue>, error out=w41:errorcluster)  [unwired: 3 in, 1 out]
  n217 = Obtain Notifier(name (unnamed)="TP" ("名称（未命名）"), notification data type=FALSE) -> (notifier out=w11:refnum<notifier>)  [unwired: 2 in, 2 out]
  n218 = while {
    tunnel: w40 -> [w389]
    tunnel: w41 -> [_]
    stop <- FALSE stop-if-true
    w376 = u16 1 items=["总磷"=1, "总氮"=2, "氨氮"=3] ("站号")
    # "试剂填充 172 \n管路清洗108\n氨氮92\n总磷131\n总磷海水147\n总氮76\n总氮海水92"
    n219 = Wait (ms)(milliseconds to wait=u32 1000 ("等待时间（毫秒）")) -> ()  [unwired: 1 out]
    n220 = global read "VAR总磷氨氮全局变量.vi" "状态告警区"() -> (w377:T4)
    n221 = Bundle By Name(cluster=cluster{"命令":string, "data":variant} {"命令"="", "data"=variant} ("元素"), "命令"="读状态告警区", "data"=w376) -> (w391:cluster{"命令":string, "data":variant})
    n222 = Unbundle By Name(w377) -> ("系统时间"=w384:timestamp)
    n223 = Get Date/Time In Seconds() -> (seconds since 1Jan1904=w383:timestamp)
    n224 = Subtract(x=w383, y=w384) -> (x-y=w382:dbl)
    n225 = Enqueue Element(queue=w389, element=w391) -> (queue out=w385:refnum<queue>)  [unwired: 2 in, 2 out]
    n226 = Absolute Value(x=w382) -> (abs(x)=w381:dbl)
    n227 = Bundle By Name(cluster=cluster{"命令":string, "data":variant} {"命令"="", "data"=variant} ("元素"), "命令"="读测量数据区", "data"=w376) -> (w387:cluster{"命令":string, "data":variant})
    n228 = global read "VAR总磷氨氮全局变量.vi" "通讯状态"() -> (w374:bool)
    n229 = Greater Or Equal?(x=w381, y=120.0) -> (x >= y?=w379:bool)
    n230 = And(x=w374, y=w379) -> (x .and. y?=w375:bool)
    n231 = Enqueue Element(queue=w385, element=w387) -> (queue out=w378:refnum<queue>)  [unwired: 2 in, 2 out]
    n232 = case shown="真" w375 {
      tunnel: w378 -> [_ w396]
      frame False {
      }
      frame True {
        n233 = call "总磷氨氮启动命令.vi"("参数"=T5 {"站号"=3, "量程切换"=enum."AUTO", "控制命令"=enum."校时", "模式设置"=enum."待机", "测量间隔"=0}) -> ("启动命令"=w395:cluster{"命令":string, "data":variant})  [unwired: 10 in]
        n234 = Enqueue Element(queue=w396, element=w395) -> ()  [unwired: 2 in, 3 out]
      }
    }
  }
  n235 = while {
    tunnel: w40 -> [w405]
    tunnel: w23 -> [w404]
    tunnel: w22 -> [w403]
    tunnel: w21 -> [w402]
    tunnel: w20 -> [w401]
    tunnel: w19 -> [w400]
    tunnel: w18 -> [w399]
    tunnel: w11 -> [w398]
    tunnel: w1 -> [_]
    stop <- FALSE stop-if-true
    n236 = event shown="[1] \"质控参数设置\": 值改变" {
      selector: _ -> [_ _ _ _ _ _ _ _ _ _ _ _ _ _ _ _ _ _ _]
      dyn-events: _ -> [_ _ _ _ _ _ _ _ _ _ _ _ _ _ _ _ _ _ _]
      timeout: _ -> [_ _ _ _ _ _ _ _ _ _ _ _ _ _ _ _ _ _ _]
      tunnel: w405 -> [_ _ _ w450 _ w475 w482 _ _ _ _ _ _ _ _ _ _ _ _]
      tunnel: w404 -> [_ _ _ _ _ _ _ _ _ _ _ _ _ w572 _ w592 w601 _ _]
      tunnel: w403 -> [_ _ _ _ _ _ _ _ _ _ _ _ _ w570 _ w590 w603 w611 w618]
      tunnel: w402 -> [_ _ _ _ _ _ _ _ _ _ _ _ _ w571 _ w591 w602 _ _]
      tunnel: w401 -> [_ _ _ _ _ _ _ _ _ _ _ _ _ w566 _ _ _ _ _]
      tunnel: w400 -> [_ _ _ _ _ _ _ _ _ _ _ _ _ _ _ w586 _ _ _]
      tunnel: w399 -> [_ _ _ _ _ _ _ _ _ _ _ _ _ _ _ _ _ w609 _]
      tunnel: w398 -> [_ _ _ _ _ _ w478 _ _ _ _ _ _ _ _ _ _ _ _]
      event Timeout {
        n237 = event-data() -> ()  [unwired: 1 in, 3 out]
      }
      event "质控参数设置": Value Change {
        n238 = event-data() -> ()  [unwired: 1 in, 6 out]
        n239 = global read "总磷断电保存全局变量.vi" "质控参数设置"() -> (w407:T20)
        n240 = call "总磷质控参数设置.vi"("质控参数设置"=w407) -> ("输出簇"=w408:T21)  [unwired: 10 in]
        n241 = Unbundle By Name(w408) -> ("确定"=w409:bool)
        n242 = case shown="真" w409 {
          tunnel: w408 -> [_ w411]
          tunnel: w407 -> [_ w410]
          frame False {
          }
          frame True {
            n243 = flat-sequence {
              tunnel: w411 -> [w418]
              tunnel: w410 -> [w412]
              frame #0 {
                n244 = Unbundle By Name(w418) -> ("跨度值"=w414:dbl, "零点标准液浓度"=w415:dbl, "跨度标准液浓度"=w416:dbl, "标准液标准浓度"=w417:dbl)
                n245 = Bundle By Name(cluster=w412, "跨度值"=w414, "零点标准液浓度"=w415, "跨度标准液浓度"=w416, "标准液标准浓度"=w417) -> (w413:T20)
                n246 = global write "总磷断电保存全局变量.vi" "质控参数设置"(w413) -> ()
              }
              frame #1 {
                n247 = call <vilib>:"Application Directory.vi"() -> ("Application Directory"=w432:path)
                n248 = Build Path(base path=w432, name or relative path="data\\sys.ini" ("名称或相对路径")) -> (appended path=w430:path)
                n249 = call <vilib>:"Open Config Data.vi"("configuration file path"=w430) -> ("error out"=w426:errorcluster, "refnum"=w429:T18)  [unwired: 8 in, 1 out]
                n250 = vi-ref "斯坦道仪器.lvlib:总磷断电保存全局变量.vi"() -> (w428:refnum<vi>)
                n251 = call <userlib>:"Write Panel to INI__ogtk.vi"("error in (no error)"=w426, "VI ref"=w428, "refnum"=w429) -> ("error out"=w425:errorcluster, "refnum out"=w427:T18)  [unwired: 7 in]
                n252 = call <vilib>:"Close Config Data.vi"("error in (no error)"=w425, "refnum"=w427) -> ("error out"=w420:errorcluster, "file path"=w419:path)  [unwired: 8 in]
                n253 = Open/Create/Replace File(file path (use dialog)=w419, error in=w420) -> (refnum out=w423:refnum<file>, error out=w424:errorcluster)  [unwired: 4 in, 1 out]
                n254 = Flush File(refnum=w423, error in=w424) -> (refnum out=w422:refnum<file>, error out=w421:errorcluster)
                n255 = Close File(refnum=w422, error in=w421) -> ()  [unwired: 2 out]
              }
            }
          }
        }
      }
      event "总磷自动测试量程配置": Value Change {
        n256 = event-data() -> ()  [unwired: 1 in, 6 out]
        n257 = flat-sequence {
          frame #0 {
            n258 = global write "总磷断电保存全局变量.vi" "总磷自动测试量程配置"("总磷自动测试量程配置") -> ()
          }
          frame #1 {
            n259 = call <vilib>:"Application Directory.vi"() -> ("Application Directory"=w447:path)
            n260 = Build Path(base path=w447, name or relative path="data\\sys.ini" ("名称或相对路径")) -> (appended path=w445:path)
            n261 = call <vilib>:"Open Config Data.vi"("configuration file path"=w445) -> ("error out"=w441:errorcluster, "refnum"=w444:T18)  [unwired: 8 in, 1 out]
            n262 = vi-ref "斯坦道仪器.lvlib:总磷断电保存全局变量.vi"() -> (w443:refnum<vi>)
            n263 = call <userlib>:"Write Panel to INI__ogtk.vi"("error in (no error)"=w441, "VI ref"=w443, "refnum"=w444) -> ("error out"=w440:errorcluster, "refnum out"=w442:T18)  [unwired: 7 in]
            n264 = call <vilib>:"Close Config Data.vi"("error in (no error)"=w440, "refnum"=w442) -> ("error out"=w435:errorcluster, "file path"=w434:path)  [unwired: 8 in]
            n265 = Open/Create/Replace File(file path (use dialog)=w434, error in=w435) -> (refnum out=w438:refnum<file>, error out=w439:errorcluster)  [unwired: 4 in, 1 out]
            n266 = Flush File(refnum=w438, error in=w439) -> (refnum out=w437:refnum<file>, error out=w436:errorcluster)
            n267 = Close File(refnum=w437, error in=w436) -> ()  [unwired: 2 out]
          }
        }
      }
      event "手动启动": Value Change {
        n268 = event-data() -> ()  [unwired: 1 in, 6 out]
        n269 = call "总磷氨氮启动参数对话框.vi"() -> ("确认"=w448:bool, "元素"=w449:cluster{"命令":string, "data":variant})  [unwired: 10 in]
        n270 = case shown="真" w448 {
          tunnel: w450 -> [_ w452]
          tunnel: w449 -> [_ w451]
          frame False {
          }
          frame True {
            n271 = Enqueue Element(queue=w452, element=w451) -> ()  [unwired: 2 in, 3 out]
          }
        }
      }
      event "定时启动": Mouse Down {
        n272 = event-data() -> ()  [unwired: 1 in, 6 out]
        n273 = flat-sequence {
          frame #0 {
            n274 = global read "总磷断电保存全局变量.vi" "定时控制"() -> (w453:T7)
            n275 = call "周期设置.vi"("定时控制参数输入"=w453) -> ("定时控制参数输出"=w454:T7)  [unwired: 10 in]
            n276 = global write "总磷断电保存全局变量.vi" "定时控制"(w454) -> ()
          }
          frame #1 {
            n277 = call <vilib>:"Application Directory.vi"() -> ("Application Directory"=w468:path)
            n278 = Build Path(base path=w468, name or relative path="data\\sys.ini" ("名称或相对路径")) -> (appended path=w466:path)
            n279 = call <vilib>:"Open Config Data.vi"("configuration file path"=w466) -> ("error out"=w462:errorcluster, "refnum"=w465:T18)  [unwired: 8 in, 1 out]
            n280 = vi-ref "斯坦道仪器.lvlib:总磷断电保存全局变量.vi"() -> (w464:refnum<vi>)
            n281 = call <userlib>:"Write Panel to INI__ogtk.vi"("error in (no error)"=w462, "VI ref"=w464, "refnum"=w465) -> ("error out"=w461:errorcluster, "refnum out"=w463:T18)  [unwired: 7 in]
            n282 = call <vilib>:"Close Config Data.vi"("error in (no error)"=w461, "refnum"=w463) -> ("error out"=w456:errorcluster, "file path"=w455:path)  [unwired: 8 in]
            n283 = Open/Create/Replace File(file path (use dialog)=w455, error in=w456) -> (refnum out=w459:refnum<file>, error out=w460:errorcluster)  [unwired: 4 in, 1 out]
            n284 = Flush File(refnum=w459, error in=w460) -> (refnum out=w458:refnum<file>, error out=w457:errorcluster)
            n285 = Close File(refnum=w458, error in=w457) -> ()  [unwired: 2 out]
          }
        }
      }
      event "单步测试": Value Change {
        w470 = u16 1 items=["总磷"=1, "氨氮"=3] ("站号")
        n286 = event-data() -> ()  [unwired: 1 in, 6 out]
        n287 = Bundle("站号"=w470, "总磷氨氮调试"="总磷氨氮调试") -> (w469:cluster{"站号":u16, "总磷氨氮调试":u16[]})  [unwired: 1 in]
        n288 = Bundle By Name(cluster=cluster{"命令":string, "data":variant} {"命令"="", "data"=variant} ("元素"), "命令"="debug", "data"=w469) -> (w472:cluster{"命令":string, "data":variant})
        n289 = Enqueue Element(queue=w475, element=w472) -> ()  [unwired: 2 in, 3 out]
      }
      event "停止": Value Change {
        n290 = event-data() -> ()  [unwired: 1 in, 6 out]
        n291 = Enqueue Element(queue=w482, element=cluster{"命令":string, "data":variant} {"命令"="启动", "data"=variant(cluster{"站号":u16, "控制命令输出":u16[]} {"站号"=1, "控制命令输出"=[2816]})} ("元素")) -> (queue out=w479:refnum<queue>)  [unwired: 2 in, 2 out]
        n292 = Cancel Notification(0:w478) -> (8:w477:refnum<notifier>)  [unwired: 1 in, 2 out]
        n293 = Send Notification(notification=TRUE ("通知"), notifier=w477) -> ()  [unwired: 1 in, 2 out]
        n294 = Enqueue Element(queue=w479, element=cluster{"命令":string, "data":variant} {"命令"="启动", "data"=variant(cluster{"站号":u16, "控制命令输出":u16[]} {"站号"=2, "控制命令输出"=[2816]})} ("元素")) -> ()  [unwired: 2 in, 3 out]
      }
      event "设置": Value Change {
        n295 = event-data() -> ()  [unwired: 1 in, 6 out]
        n296 = property on="窗格" class="Pane"("Origin"=T10 {"Horizontal"=0, "Vertical"=628} ("原点")) -> ()  [unwired: 2 in, 2 out]
      }
      event "返回": Value Change {
        n297 = event-data() -> ()  [unwired: 1 in, 6 out]
        n298 = property on="窗格" class="Pane"("Origin"=T10 {"Horizontal"=0, "Vertical"=0} ("原点")) -> ()  [unwired: 2 in, 2 out]
      }
      event "标液浓度1", "测量吸光度1", "测量吸光度2", "标液浓度2", "测量吸光度3", "标液浓度3", "测量吸光度4", "标液浓度4", "测量吸光度5", "标液浓度5", "样品1启用", "样品3启用", "样品4启用", "样品5启用", "样品2启用", "模型", "method", "精度": Value Change {
        n299 = event-data() -> ()  [unwired: 1 in, 6 out]
        n300 = flat-sequence {
          frame #0 {
            n301 = Replace Array Subset(array=dbl[] [0.0, 0.0, 0.0, 0.0, 0.0] ("数组"), new element #1="标液浓度1", new element #2="标液浓度2", new element #3="标液浓度3", new element #4="标液浓度4", new element #5="标液浓度5") -> (w520:dbl[])  [unwired: 5 in]
            n302 = Replace Array Subset(array=dbl[] [0.0, 0.0, 0.0, 0.0, 0.0] ("数组"), new element #1="测量吸光度1", new element #2="测量吸光度2", new element #3="测量吸光度3", new element #4="测量吸光度4", new element #5="测量吸光度5") -> (w519:dbl[])  [unwired: 5 in]
            n303 = Replace Array Subset(array=bool[] [FALSE, FALSE, FALSE, FALSE, FALSE] ("数组"), new element #1="样品1启用", new element #2="样品2启用", new element #3="样品3启用", new element #4="样品4启用", new element #5="样品5启用") -> (w518:bool[])  [unwired: 5 in]
            n304 = call "线性公式.vi"("精度"="精度", "模型"="模型", "method"="method", "启用"=w518, "监测浓度"=w519, "标液浓度"=w520) -> ("XY图"=w495:cluster{"X Values":dbl[], "Y Values":dbl[]}[], "r^2"=w496:dbl, "拟合方程"=w497:string)  [unwired: 3 in]
            "XY图" <- w495
            "拟合公式" <- w497
            "r^2" <- w496
            n305 = global read "总磷断电保存全局变量.vi" "曲线模型"() -> (w517:T19)
            n306 = local read "样品1 F0"() -> (w494:dbl)
            n307 = local read "样品1 F1"() -> (w493:dbl)
            n308 = local read "样品2 F0"() -> (w492:dbl)
            n309 = local read "样品2 F1"() -> (w491:dbl)
            n310 = local read "样品3 F0"() -> (w490:dbl)
            n311 = local read "样品3 F1"() -> (w489:dbl)
            n312 = local read "样品4 F0"() -> (w488:dbl)
            n313 = local read "样品4 F1"() -> (w487:dbl)
            n314 = local read "样品5 F0"() -> (w486:dbl)
            n315 = local read "样品5 F1"() -> (w485:dbl)
            n316 = Bundle By Name(cluster=w517, "标液浓度1"="标液浓度1", "标液浓度2"="标液浓度2", "标液浓度3"="标液浓度3", "标液浓度4"="标液浓度4", "标液浓度5"="标液浓度5", "测量吸光度1"="测量吸光度1", "测量吸光度2"="测量吸光度2", "测量吸光度3"="测量吸光度3", "测量吸光度4"="测量吸光度4", "测量吸光度5"="测量吸光度5", "样品1启用"="样品1启用", "样品2启用"="样品2启用", "样品3启用"="样品3启用", "样品4启用"="样品4启用", "样品5启用"="样品5启用", "模型"="模型", "method"="method", "精度"="精度", "拟合公式"=w497, "r^2"=w496, "XY图"=w495, "样品1 F0"=w494, "样品1 F1"=w493, "样品2 F0"=w492, "样品2 F1"=w491, "样品3 F0"=w490, "样品3 F1"=w489, "样品4 F0"=w488, "样品4 F1"=w487, "样品5 F0"=w486, "样品5 F1"=w485) -> (w516:T19)
            n317 = global write "总磷断电保存全局变量.vi" "曲线模型"(w516) -> ()
          }
          frame #1 {
            n318 = call <vilib>:"Application Directory.vi"() -> ("Application Directory"=w537:path)
            n319 = Build Path(base path=w537, name or relative path="data\\sys.ini" ("名称或相对路径")) -> (appended path=w535:path)
            n320 = call <vilib>:"Open Config Data.vi"("configuration file path"=w535) -> ("error out"=w532:errorcluster, "refnum"=w534:T18)  [unwired: 8 in, 1 out]
            n321 = vi-ref "斯坦道仪器.lvlib:总磷断电保存全局变量.vi"() -> (w524:refnum<vi>)
            n322 = call <userlib>:"Write Panel to INI__ogtk.vi"("error in (no error)"=w532, "VI ref"=w524, "refnum"=w534) -> ("error out"=w531:errorcluster, "refnum out"=w533:T18)  [unwired: 7 in]
            n323 = call <vilib>:"Close Config Data.vi"("error in (no error)"=w531, "refnum"=w533) -> ("error out"=w526:errorcluster, "file path"=w525:path)  [unwired: 8 in]
            n324 = Open/Create/Replace File(file path (use dialog)=w525, error in=w526) -> (refnum out=w529:refnum<file>, error out=w530:errorcluster)  [unwired: 4 in, 1 out]
            n325 = Flush File(refnum=w529, error in=w530) -> (refnum out=w528:refnum<file>, error out=w527:errorcluster)
            n326 = Close File(refnum=w528, error in=w527) -> ()  [unwired: 2 out]
          }
        }
      }
      event "样品1 F0", "样品1 F1", "样品2 F1", "样品2 F0", "样品3 F1", "样品3 F0", "样品4 F0", "样品4 F1", "样品5 F1", "样品5 F0": Value Change {
        n327 = event-data() -> ()  [unwired: 1 in, 6 out]
        n328 = formula code="E=log(F0/F1);"("F0"="样品5 F0", "F1"="样品5 F1") -> ("E"=w538:dbl)
        n329 = formula code="E=log(F0/F1);"("F0"="样品4 F0", "F1"="样品4 F1") -> ("E"=w539:dbl)
        n330 = formula code="E=log(F0/F1);"("F0"="样品3 F0", "F1"="样品3 F1") -> ("E"=w540:dbl)
        n331 = formula code="E=log(F0/F1);"("F0"="样品2 F0", "F1"="样品2 F1") -> ("E"=w541:dbl)
        n332 = formula code="E=log(F0/F1);"("F0"="样品1 F0", "F1"="样品1 F1") -> ("E"=w542:dbl)
        n333 = property on="测量吸光度5" class="DigNum (严格)"("Val(Sgnl)"=w538) -> ()  [unwired: 2 in, 2 out]
        n334 = property on="测量吸光度4" class="DigNum (严格)"("Val(Sgnl)"=w539) -> ()  [unwired: 2 in, 2 out]
        n335 = property on="测量吸光度3" class="DigNum (严格)"("Val(Sgnl)"=w540) -> ()  [unwired: 2 in, 2 out]
        n336 = property on="测量吸光度2" class="DigNum (严格)"("Val(Sgnl)"=w541) -> ()  [unwired: 2 in, 2 out]
        n337 = property on="测量吸光度1" class="DigNum (严格)"("Val(Sgnl)"=w542) -> ()  [unwired: 2 in, 2 out]
      }
      event "标液浓度1", "标液浓度2", "标液浓度3", "标液浓度4", "标液浓度5", "样品1 F0", "样品1 F1", "样品2 F1", "样品2 F0", "样品3 F1", "样品3 F0", "样品4 F0", "样品4 F1", "样品5 F0", "样品5 F1", "精度", "公式.X^2", "公式.X", "公式.b", "量程切换阈值.阈值", "量程切换阈值.标液浓度", "备用系数.量程上限", "备用系数.量程下限", "备用系数.检出限", "备用系数.精度": Mouse Down {
        n338 = event-data() -> ("CtlRef"=w556:refnum<vi>)  [unwired: 1 in, 5 out]
        n339 = property class="DigNum (严格)"(reference=w556) -> (reference out=w554:refnum<vi>, "Value"=w555:dbl)  [unwired: 1 in, 1 out]
        n340 = call "数字键盘.vi"("OldNumber"=w555) -> ("NewNumber"=w553:dbl)
        n341 = property class="DigNum (严格)"(reference=w554, "Val(Sgnl)"=w553) -> ()  [unwired: 1 in, 2 out]
      }
      event "测量吸光度1", "测量吸光度2", "测量吸光度3", "测量吸光度4", "测量吸光度5": Mouse Down {
        n342 = event-data() -> ("CtlRef"=w560:refnum<vi>)  [unwired: 1 in, 7 out]
        n343 = property class="DigNum (严格)"(reference=w560) -> (reference out=w561:refnum<vi>, "Value"=w558:dbl)  [unwired: 1 in, 1 out]
        n344 = call "数字键盘.vi"("OldNumber"=w558) -> ("NewNumber"=w559:dbl)
        n345 = property class="DigNum (严格)"(reference=w561, "Val(Sgnl)"=w559) -> ()  [unwired: 1 in, 2 out]
        n346 = Not Equal?(x=w559, y=w558) -> (x != y?=w557:bool)
        n347 = case shown="真" w557 {
          frame False {
          }
          frame True {
            w562 = 0.0 ("样品1 F0")
            n348 = local write "样品1 F0"(w562) -> ()
            n349 = local write "样品1 F1"(w562) -> ()
            n350 = local write "样品2 F1"(w562) -> ()
            n351 = local write "样品2 F0"(w562) -> ()
            n352 = local write "样品3 F1"(w562) -> ()
            n353 = local write "样品3 F0"(w562) -> ()
            n354 = local write "样品4 F0"(w562) -> ()
            n355 = local write "样品4 F1"(w562) -> ()
            n356 = local write "样品5 F1"(w562) -> ()
            n357 = local write "样品5 F0"(w562) -> ()
          }
        }
      }
      event "读公式": Value Change {
        n358 = event-data() -> ()  [unwired: 1 in, 6 out]
        n359 = property class="Enum (严格)"(reference=w570) -> ("Value"=w569:enum16{"总磷", "总氮"})  [unwired: 1 in, 2 out]
        n360 = property class="Enum (严格)"(reference=w571) -> ("Value"=w568:enum16{"水样测量", "空白核查", "跨度核查", "标样核查", "加标回收"})  [unwired: 1 in, 2 out]
        n361 = property class="Enum (严格)"(reference=w572) -> ("Value"=w567:enum16{"低量程", "高量程"})  [unwired: 1 in, 2 out]
        n362 = call "总磷氨氮公式读取.vi"("量程"=w567, "测量模式"=w568, "测量参数"=w569) -> ("error out"=w564:errorcluster, "公式"=w565:cluster{"X^2":dbl, "X":dbl, "b":dbl})  [unwired: 7 in]
        n363 = property class="Clust (严格)"(reference=w566, "Value"=w565) -> ()  [unwired: 1 in, 2 out]
        n364 = case shown="错误" w564 {
          tunnel: ["读取成功" ("消息") "读取失败" ("消息")] -> w563
          frame No Error {
          }
          frame Error {
          }
        }
        n365 = One Button Dialog(message=w563) -> ()  [unwired: 1 in, 1 out]
      }
      event "写公式": Value Change {
        n366 = event-data() -> ()  [unwired: 1 in, 6 out]
        n367 = call "总磷氨氮公式写入.vi"("公式"="公式", "量程"="量程下拉列表", "测量模式"="测量模式下拉列表", "测量参数"="参数下拉列表") -> ("error out"=w577:errorcluster)  [unwired: 7 in]
        n368 = case shown="无错误" w577 {
          tunnel: ["写入成功" ("消息") "写入失败" ("消息")] -> w578
          frame No Error {
          }
          frame Error {
          }
        }
        n369 = One Button Dialog(message=w578) -> ()  [unwired: 1 in, 1 out]
      }
      event "量程切换阈值读取": Value Change {
        n370 = event-data() -> ()  [unwired: 1 in, 6 out]
        n371 = property class="Enum (严格)"(reference=w590) -> ("Value"=w589:enum16{"总磷", "总氮"})  [unwired: 1 in, 2 out]
        n372 = property class="Enum (严格)"(reference=w591) -> ("Value"=w588:enum16{"水样测量", "空白核查", "跨度核查", "标样核查", "加标回收"})  [unwired: 1 in, 2 out]
        n373 = property class="Enum (严格)"(reference=w592) -> ("Value"=w587:enum16{"低量程", "高量程"})  [unwired: 1 in, 2 out]
        n374 = call "总磷氨氮量程读取.vi"("量程"=w587, "测量模式"=w588, "测量参数"=w589) -> ("error out"=w583:errorcluster, "量程切换阈值"=w585:cluster{"阈值":dbl, "标液浓度":dbl})  [unwired: 7 in]
        n375 = property class="Clust (严格)"(reference=w586, "Value"=w585) -> ()  [unwired: 1 in, 2 out]
        n376 = case shown="错误" w583 {
          tunnel: ["读取成功" ("消息") "读取失败" ("消息")] -> w584
          frame No Error {
          }
          frame Error {
          }
        }
        n377 = One Button Dialog(message=w584) -> ()  [unwired: 1 in, 1 out]
      }
      event "量程切换阈值写入": Value Change {
        n378 = event-data() -> ()  [unwired: 1 in, 6 out]
        n379 = property class="Enum (严格)"(reference=w603) -> ("Value"=w600:enum16{"总磷", "总氮"})  [unwired: 1 in, 2 out]
        n380 = property class="Enum (严格)"(reference=w602) -> ("Value"=w599:enum16{"水样测量", "空白核查", "跨度核查", "标样核查", "加标回收"})  [unwired: 1 in, 2 out]
        n381 = property class="Enum (严格)"(reference=w601) -> ("Value"=w598:enum16{"低量程", "高量程"})  [unwired: 1 in, 2 out]
        n382 = call "总磷氨氮量程写入.vi"("量程切换阈值"="量程切换阈值", "量程"=w598, "测量模式"=w599, "测量参数"=w600) -> ("error out"=w595:errorcluster)  [unwired: 7 in]
        n383 = case shown="无错误" w595 {
          tunnel: ["写入成功" ("消息") "写入失败" ("消息")] -> w596
          frame No Error {
          }
          frame Error {
          }
        }
        n384 = One Button Dialog(message=w596) -> ()  [unwired: 1 in, 1 out]
      }
      event "备用系数读取": Value Change {
        n385 = event-data() -> ()  [unwired: 1 in, 6 out]
        n386 = property class="Enum (严格)"(reference=w611) -> ("Value"=w610:enum16{"总磷", "总氮"})  [unwired: 1 in, 2 out]
        n387 = call "总磷氨氮备用系数读取.vi"("测量参数"=w610) -> ("error out"=w606:errorcluster, "备用系数"=w608:T2)  [unwired: 9 in]
        n388 = property class="Clust (严格)"(reference=w609, "Value"=w608) -> ()  [unwired: 1 in, 2 out]
        n389 = case shown="错误" w606 {
          tunnel: ["读取成功" ("消息") "读取失败" ("消息")] -> w607
          frame No Error {
          }
          frame Error {
          }
        }
        n390 = One Button Dialog(message=w607) -> ()  [unwired: 1 in, 1 out]
      }
      event "备用系数写入": Value Change {
        n391 = event-data() -> ()  [unwired: 1 in, 6 out]
        n392 = property class="Enum (严格)"(reference=w618) -> ("Value"=w617:enum16{"总磷", "总氮"})  [unwired: 1 in, 2 out]
        n393 = call "总磷氨氮备用系数写入.vi"("备用系数"="备用系数", "测量参数"=w617) -> ("error out"=w614:errorcluster)  [unwired: 9 in]
        n394 = case shown="无错误" w614 {
          tunnel: ["写入成功" ("消息") "写入失败" ("消息")] -> w615
          frame No Error {
          }
          frame Error {
          }
        }
        n395 = One Button Dialog(message=w615) -> ()  [unwired: 1 in, 1 out]
      }
    }
  }
